vi "Alladio Tool.vi"() -> ()   [LabVIEW 2021]
doc: "Aplicación para evaluación de aparatos que usen el protocolo GEA2."
uses:
  Common/LabVIEW GEA2 Toolkit/GEA3/type defs/Data In.ctl
  Common/LabVIEW GEA2 Toolkit/GEA3/type defs/Source_Destination.ctl
  Common/LabVIEW GEA2 Toolkit/GEA3/type defs/ERD Write Data In.ctl
  Common/LabVIEW GEA2 Toolkit/GEA3/type defs/Data Type.ctl
  Common/LabVIEW GEA2 Toolkit/GEA3/type defs/ERD Read Data Out.ctl
  Common/LabVIEW GEA2 Toolkit/GEA3/type defs/ERD Read Data In.ctl
  Common/type defs/Programming.ctl
  Common/type defs/Flash_Results.ctl
  Common/type defs/ERDList.ctl
  Common/type defs/ERD_Loop_States.ctl
  Common/type defs/Version.ctl
  Common/type defs/BootloaderVersion.ctl
  Common/LabVIEW GEA2 Toolkit/GEA3/type defs/Data Out.ctl
  Alladio Tool Suport/Type defs/ERD_Always_Show_ARG.ctl
  Alladio Tool Suport/Type defs/Data_In_Automation_Bootloader.ctl
  Alladio Tool Suport/Type defs/Table_Result_Automation_BootLoader.ctl
  Alladio Tool Suport/Automation Erds/AT_Erd_Sequence.ctl
  Alladio Tool Suport/Automation Erds/Table_Result_AT_Test.ctl
  Alladio Tool Suport/Automation Erds/AT_Sequennce_Select.ctl
  D:/Common/LabVIEW GEA2 Toolkit/source/GEA3 DLL Source/GeaCommunication.dll
  Common/LabVIEW GEA2 Toolkit/source/GEA3 DLL Source/GeaCommunication.dll
  Common/GExplorer Support/typedefs/GExplorer_Data_Cluster.ctl
  Common/type defs/ERD_Data_Loop_Control.ctl
  Common/type defs/Error_Command.ctl
  Common/type defs/Cont_Send_States.ctl
  Alladio Tool Suport/Type defs/All_Bundled_Data_ARG.ctl
  Common/type defs/CSV_File_String_Arrays.ctl
  Common/type defs/Fault Table Array.ctl
  Common/type defs/Fault_Table_Info.ctl
  Common/type defs/ERD_Loop_Control_Command.ctl
  Common/type defs/GEA2_Control_Command.ctl
  Common/LabVIEW GEA2 Toolkit/GEA3/advanced/GEA2 Message Received Event Handler.vi
  Common/LabVIEW GEA2 Toolkit/GEA3/library/GEA2_Toolkit.lvlib
panel:
  out "UI LEDS":T1
  out "ERD_Always Show":T2
  out "Message":string
  in  "EndOfCycle":bool
  in  "Board Index":u8=1 min=1 max=10 step=1
  in  "Pause(mls)":u32=100
  out "Rate":u32=100
  out "State":T3=enum."Read ERDs"
  in  "Data ON":bool=TRUE
  in  "Stop":bool
  in  "Reset":bool
  in  "Tab Control":T4(tab)=enum."Log/Programming"
  out "Personality Set":u8=1
  in  "?":u8=1
  in  "Set Personality":bool
  out "CSV File Log Path":path=path "D:/QA/Commercial 2/Dryer_Xolo/ProbandoC2_24-11-21_15-05-37.csv"
  out "Version":T5
  in  "Read ERD List":T6[](array[typedef])=[{"ERD Number"=49, "Data Type"=enum."string"}] {"ERD Number" format="%.0x"}
  in  "Read ERD":bool
  in  "Write ERD List":T7[](array[typedef])=[{"ERD Number"=49, "Data Type"=enum."string", "Data"="01"}] {"ERD Number" format="%.0x"}
  in  "Write ERD":bool
  out "Read ERD Data Out":T9[](array[typedef])=[{"ERD Number"=49, "Data"="00 00 00 16"}] {"ERD Number" format="%.0x"}
  out "Boot Loader Version":T10
  in  "GEA Inputs":T11={"Source"=229, "Destination"=192} {"Destination" format="%.0x"; "Source" format="%.0x"}
  out "ERD's de Usuario":T12
  in  "Json File Path":path
  out "ERD Out Json":cluster{"ERD Number":u16, "Data":string}[](array[cluster]) {"ERD Number" format="%.0x"}
  out "Converted Data Out":T13 {"CRC" format="%04x"; "Length" format="%02x"; "Command" format="%02x"; "Destination" format="%02x"; "Source" format="%02x"}
  in  "Send Button":bool
  in  "GEA2 Send":T14={"Source"=228, "Destination"=192, "Command"=0, "Message"=""} {"Command" format="%02x"; "Destination" format="%02x"; "Source" format="%02x"}
  in  "Exit Botloader":bool
  in  "Enum":enum16{"All", "MC", "UI"}(ring)
  in  "Entry Botloader":bool
  out "OK?":bool
  in  "Parametric":T15(ring)
  in  "Write parametric":bool
  in  "Message to send":string="04 03"
  in  "Array":T16[](array[typedef]) {"Command" format="%02x"; "Destination" format="%02x"; "Source" format="%02x"}
  in  "Start_BootLoader":bool
  out "Bootloader Results":T17
  out "GEA2 Log":string
  in  "Save Log":bool
  in  "GEA2 Log Length":i32=100000
  in  "Clear":bool
  in  "Programming":T18={"Program"=FALSE, "File Path"=path "", "Program Ind"=FALSE, "Reset Board"=FALSE, "Enter Bootloader"=FALSE, "Result"=9} {"Result" items=["ImageRejected", "BoardNotFound", "UnableToGetGeaConfiguration", "WriteToFlashNotAllowed", "ImageDownloadedSuccessfully", "ImagePresent", "WriteToFlashFailed", "EraseFailed", "CrcFailed", ""]}
  in  "ERD Default List":T20=[{"Boolean"=TRUE, "ERD Number"=1792, "ERD Nanme"="Erd_ResetCount", "Data_Type"=enum."string"}, {"Boolean"=TRUE, "ERD Number"=61467, "ERD Nanme"="Erd_MabeCommunicationRequest1Data ", "Data_Type"=enum."string"}] {"ERD Number" format="%x"}
  in  "ERD's List Ticket Testing":T20 {"ERD Number" format="%x"}
  in  "Start_Test":bool
  in  "#Executions":i32=1 min=1 step=1
  in  "Array_Test":T21 {"Time to Wait (ms)" min=100; "ERD Number" format="%.0x"}
  in  "Sequence Select":T22
  in  "Save_Auto":bool
  out "Resultados AT Test":T23
  in  "Wifi State":T24(ring)
  in  "Set Wifi State(ERD 6003)":bool
  in  "Turn on Wifi":bool
  in  "Turn off Wifi":bool
  out "Wifi Network State":string
  out "Wifi Password":string
  out "Wifi Network Name":string
  out "Mac Address":string
  in  "Get Wifi Data":bool
  out "Error Out":errorcluster
  # "Personality"
  # "Ver. 0.1"
  # "Los primeros 10 ERD's apareceran\nen los indicadores de la página \nde GEA2"
  # "Wifi State is Writing to ERD 6003 and communicating with the wifi board directly.  It will remain in the state you wrote it to until another command is recieved. \n\nOnly Write to invalid if you are testing the board in Invalid state."
  # "After turning on Wifi , wait about 30 seconds and press the Get Wifi Data button.  Network state should be 1, apmode.\n\nAll this is doing is Writing the ERD 0xF115 Service Request to request connect, or disconnect."
  # "Contact:\n\nLeonel Nieto\nleonel.nieto@mabe.com.mx"
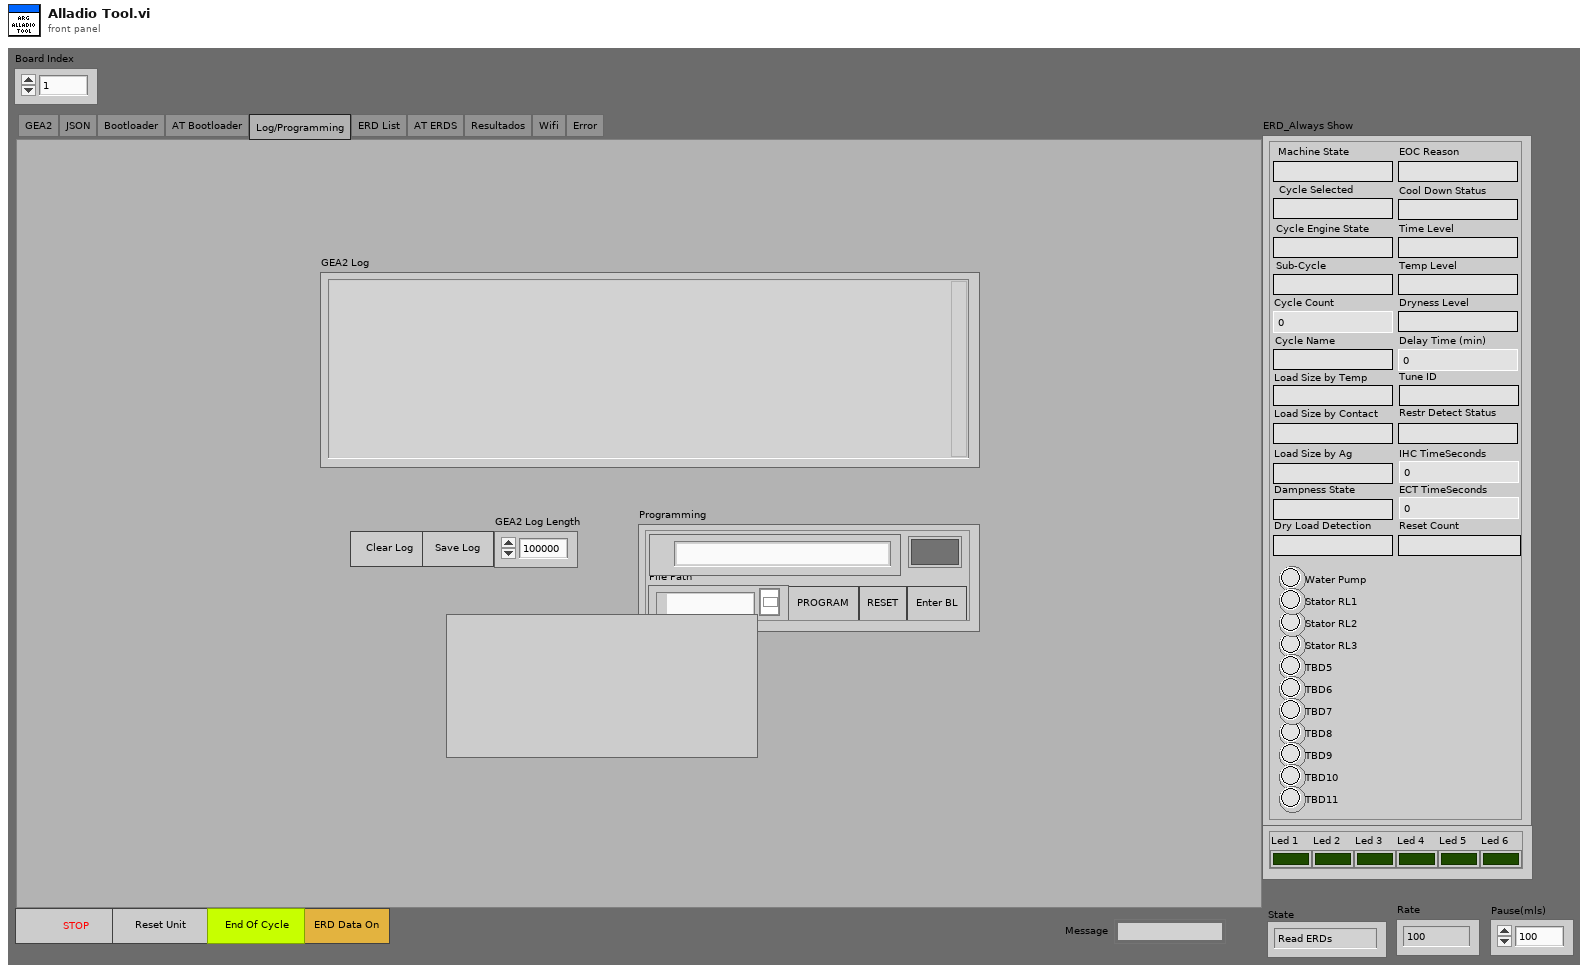
[diagram p1: front panel]
types:
  T1 = cluster{"Led 1":bool, "Led 2":bool, "Led 3":bool, "Led 4":bool, "Led 5":bool, "Led 6":bool}
  T2 = typedef "ERD_Always_Show_ARG.ctl" = cluster{"Machine State":string, "Cycle Selected":string, "Cycle Engine State":string, "Cycle Count":u32, "Temp Level":string, "Dryness Level":string, "Time Level":string, "Delay Time (min)":u16, "Sub-Cycle":string, "Cycle Name":string, "Tune ID":string, "Restr Detect Status":string, "Load Size by Contact":string, "Load Size by Temp":string, "EOC Reason":string, "Reset Count":string, "Dampness State":string, "Stator RL3":bool, "TBD5":bool, "TBD6":bool, "Water Pump":bool, "Stator RL2":bool, "Cool Down Status":string, "TBD8":bool, "TBD9":bool, "TBD10":bool, "TBD11":bool, "TBD7":bool, "Stator RL1":bool, "IHC TimeSeconds":u32, "ECT TimeSeconds ":u32, "Load Size by Ag":string, "Dry Load Detection":string}
  T3 = typedef "ERD_Loop_States.ctl" = enum16{"Init", "Build ERD Read List", "Read ERDs", "Get Version", "ERD´s User show", "Update UI", "Read Faults", "Log Data", "Pause", "Shutdown"}
  T4 = enum32{"GEA2", "JSON", "Bootloader", "AT Bootloader", "Log/Programming", "ERD List", "AT ERDS", "Resultados", "Wifi", "Error"}
  T5 = typedef "Version.ctl" = cluster{"Build Number":string, "Build Hash ":string, "Application Version":string, "Parametric Version":string, "UI App Version":string}
  T6 = typedef "ERD Read Data In.ctl" = cluster{"ERD Number":u16, "Data Type":enum16{"string", "boolean", "uint8_t", "uint16_t", "uint32_t", "uint64_t", "int8_t", "int16_t", "int32_t", "int64_t"}}
  T7 = typedef "ERD Write Data In.ctl" = cluster{"ERD Number":u16, "Data Type":T8, "Data":string}
  T8 = typedef "Data Type.ctl" = enum16{"string", "boolean", "uint8_t", "uint16_t", "uint32_t", "uint64_t", "int8_t", "int16_t", "int32_t", "int64_t"}
  T9 = typedef "ERD Read Data Out.ctl" = cluster{"ERD Number":u16, "Data":string}
  T10 = typedef "BootloaderVersion.ctl" = cluster{"UI BL Version":string, "MC BL Version":string}
  T11 = typedef "Source_Destination.ctl" = cluster{"Source":u8, "Destination":u8}
  T12 = cluster{"[0]":string, "[1]":string, "[2]":string, "[3]":string, "[4]":string, "[5]":string, "[6]":string, "[7]":string, "[8]":string, "[9]":string}
  T13 = typedef "Data Out.ctl" = cluster{"Source":u8, "Destination":u8, "Command":u8, "Length":u8, "CRC":u16, "Message":string}
  T14 = typedef "Data In.ctl" = cluster{"Source":u8, "Destination":u8, "Command":u8, "Message":string}
  T15 = enum16{"Board SKU", "Board Serial Number", "Unit SKU", "Unit Serial Number"}
  T16 = typedef "Data_In_Automation_Bootloader.ctl" = cluster{"Source":u8, "Destination":u8, "Command":u8, "Message":string, "Expected Data":string}
  T17 = typedef "Table_Result_Automation_BootLoader.ctl" = string[][]
  T18 = typedef "Programming.ctl" = cluster{"Program":bool, "File Path":path, "Program Ind":bool, "Reset Board":bool, "Enter Bootloader":bool, "Result":T19}
  T19 = typedef "Flash_Results.ctl" = i32
  T20 = typedef "ERDList.ctl" = cluster{"Boolean":bool, "ERD Number":u16, "ERD Nanme":string, "Data_Type":enum16{"string", "boolean", "uint8_t", "uint16_t", "uint32_t", "uint64_t", "int8_t", "int16_t", "int32_t", "int64_t"}}[]
  T21 = typedef "AT_Erd_Sequence.ctl" = cluster{"Accion":string, "Valor Esperado":string, "ERD Number":u16, "Data_To_Write":string, "Time to Wait (ms)":u32}[]
  T22 = typedef "AT_Sequennce_Select.ctl" = enum16{"Manual", "T361"}
  T23 = typedef "Table_Result_AT_Test.ctl" = string[][]
  T24 = enum16{"0 - OFF", "1 - App Mode", "2 - Connecting", "3 - Connected", "4 - Connected Off", "5 - Scanning", "6 - Reconnecting", "255 - Invalid"}
  T25 = typedef "All_Bundled_Data_ARG.ctl" = cluster{"Version":T5, "Personality Set":u8, "CSV File String Arrays":T26, "Fault Table Array ":T27, "ERD_Always Show":T2, "UI LEDS":cluster{"Led 1":bool, "Led 2":bool, "Led 3":bool, "Led 4":bool, "Led 5":bool, "Led 6":bool}, "Boot Loader Version":T10}
  T26 = typedef "CSV_File_String_Arrays.ctl" = cluster{"ERD Number Array":string[], "ERD Name Array":string[], "ERD Converted String Data":string[]}
  T27 = typedef "Fault Table Array.ctl" = T28[]
  T28 = typedef "Fault_Table_Info.ctl" = cluster{"Cycle Count":u32, " Runtime (min) ":u32, "Fault Status":string, "Fault ID":string, "Fault Count":u16}
  T29 = typedef "Cont_Send_States.ctl" = enum16{"Run", "Shutdown"}
  T30 = typedef "ERD_Data_Loop_Control.ctl" = cluster{"Data":variant, "State":T3}
  T31 = typedef "Error_Command.ctl" = enum16{"Initialize", "Handle Errors", "Report Errors"}
  T32 = typedef "GExplorer_Data_Cluster.ctl" = cluster{"Data":variant, "State":enum16{"Add to Log", "Clear", "Shutdown"}}
  T33 = enum8{"Enabled", "Disabled", "Disabled and Grayed Out"}
  T34 = typedef "GEA2_Control_Command.ctl" = enum16{"Initialize", "Shutdown"}
  T35 = typedef "ERD_Loop_Control_Command.ctl" = enum16{"Initialize", "Shutdown"}
  T36 = typedef "ERD_Loop_States_JL.ctl" = enum16{"Init", "Build ERD Read List", "Read ERDs", "Get Version", "ERD´s User show", "Update UI", "Read Faults", "Log Data", "Pause", "Shutdown"}
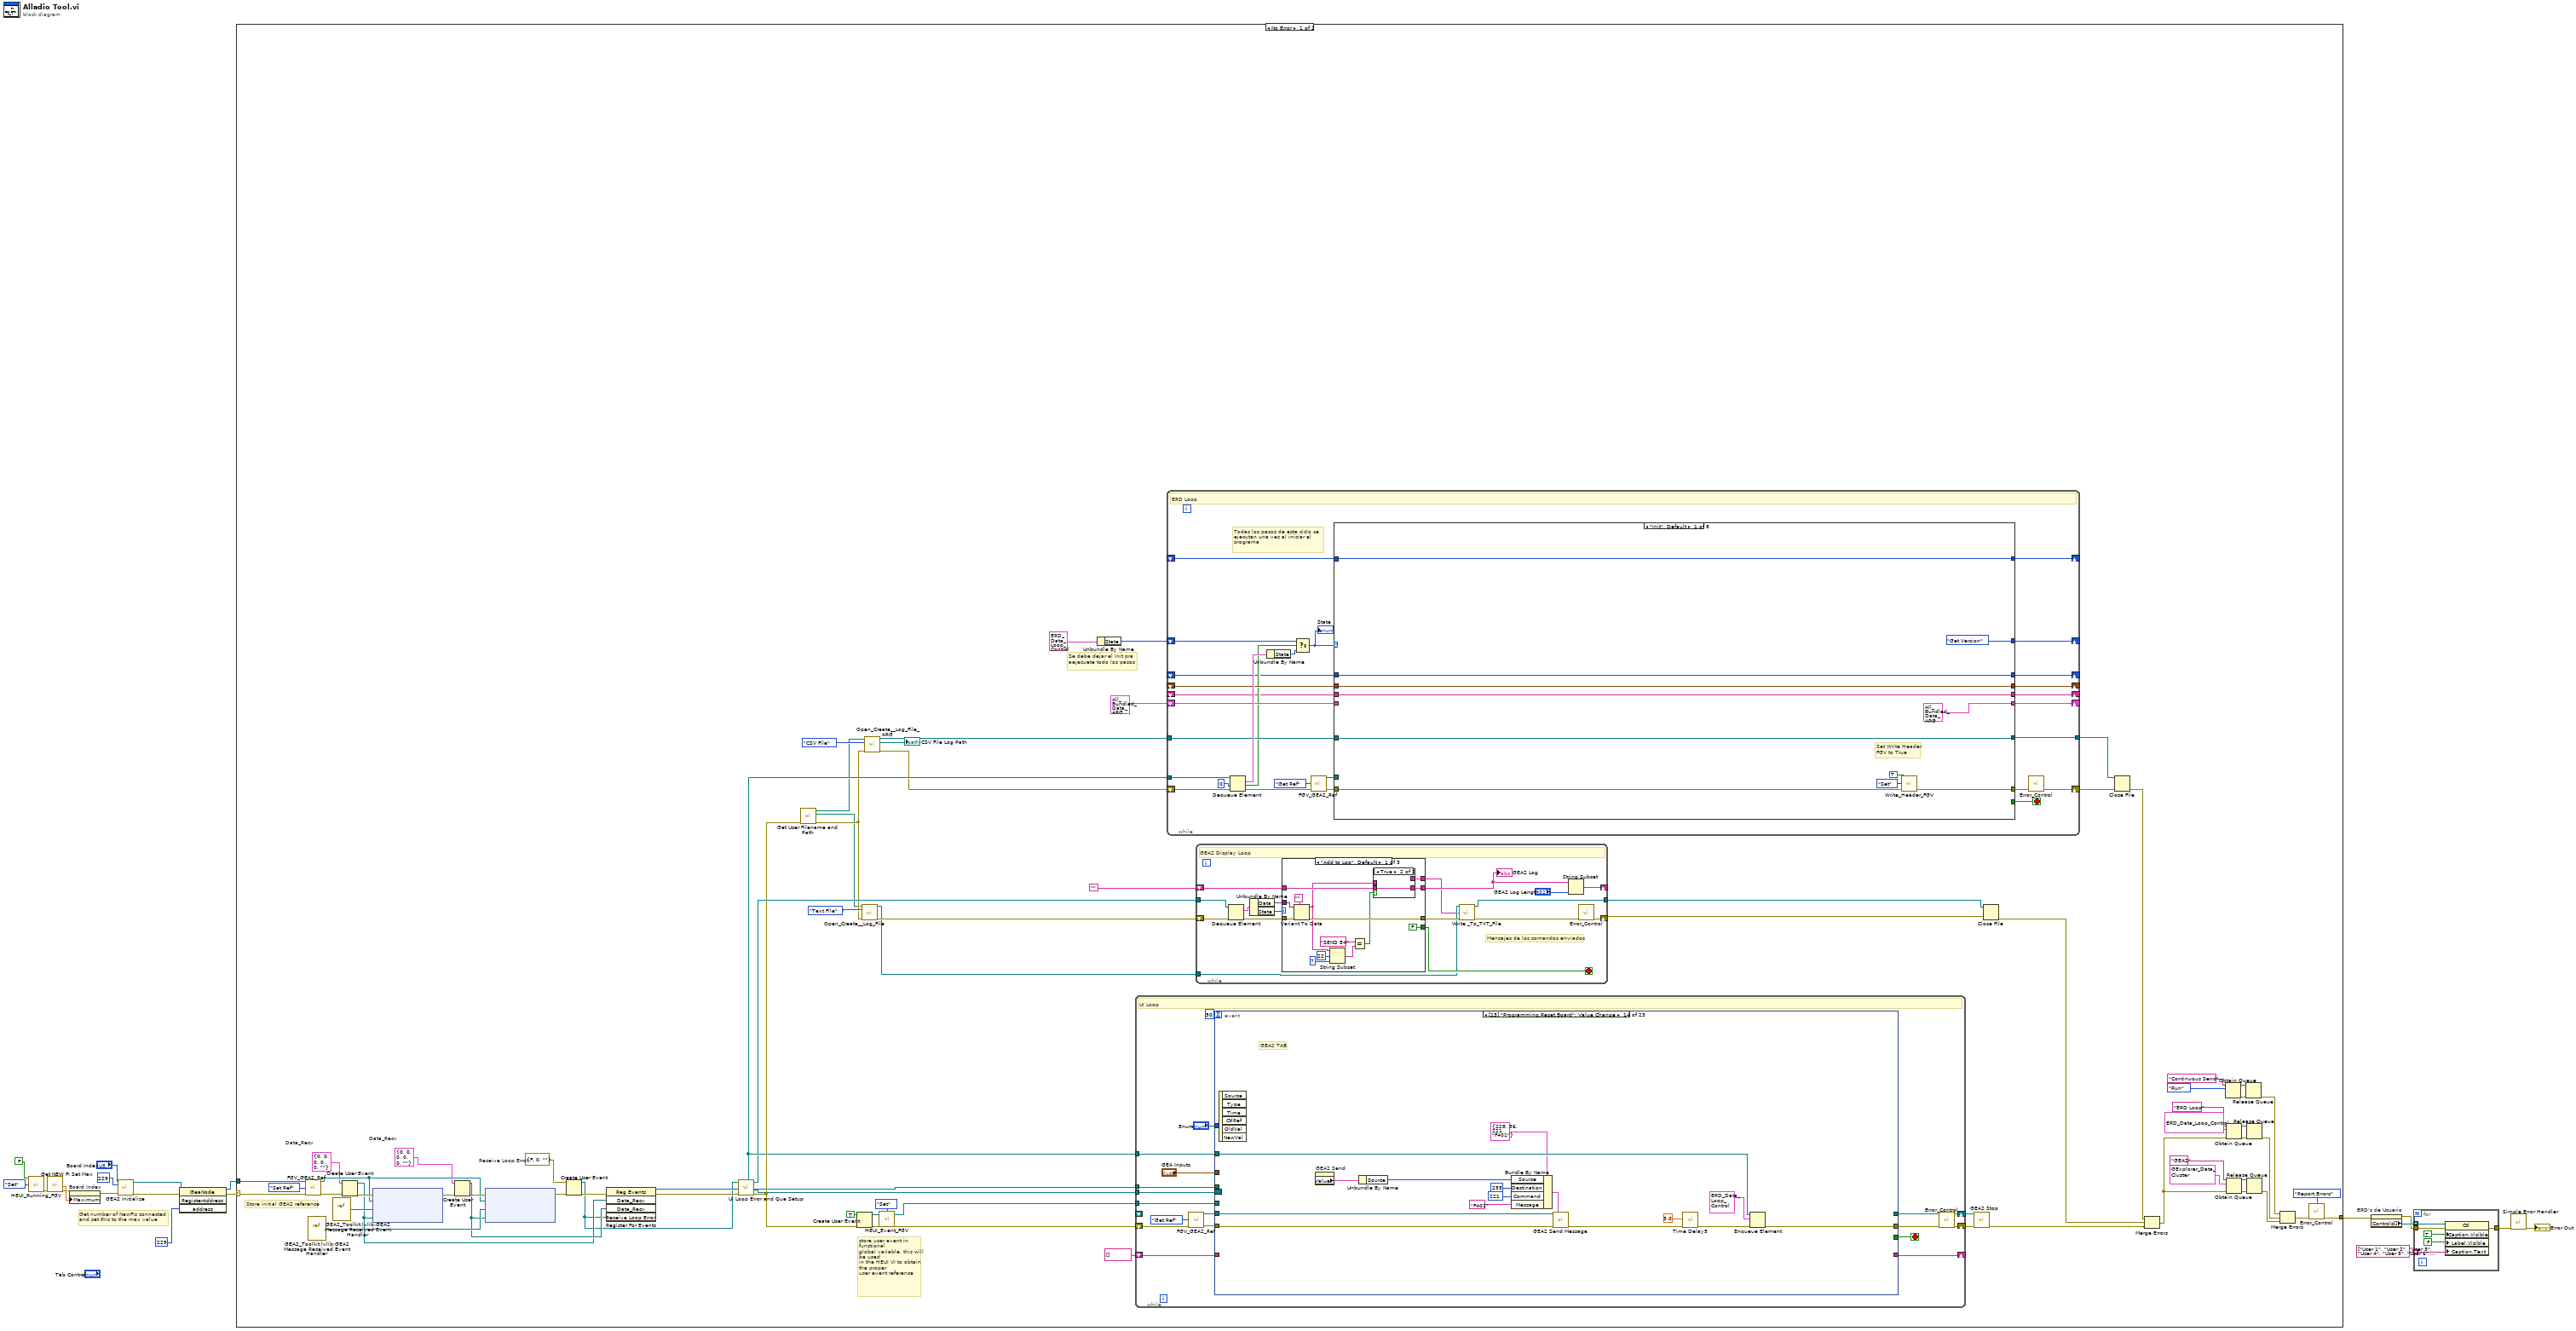
[diagram p0: block diagram]
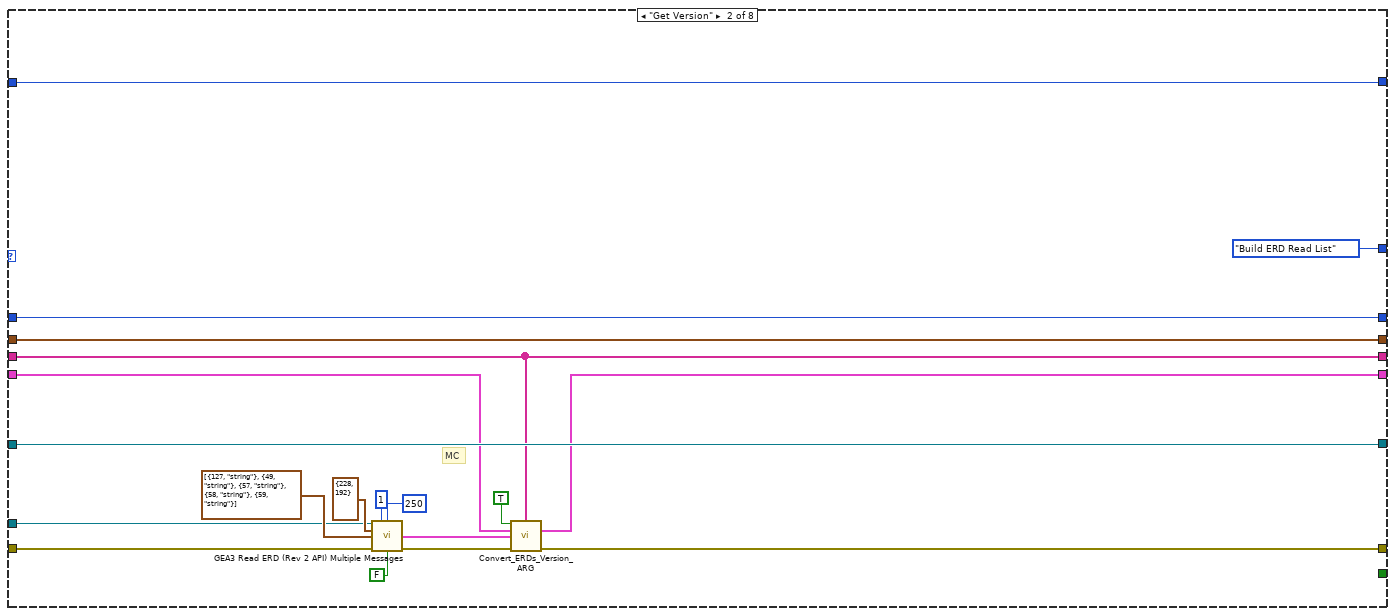
[diagram p2: hidden frame]
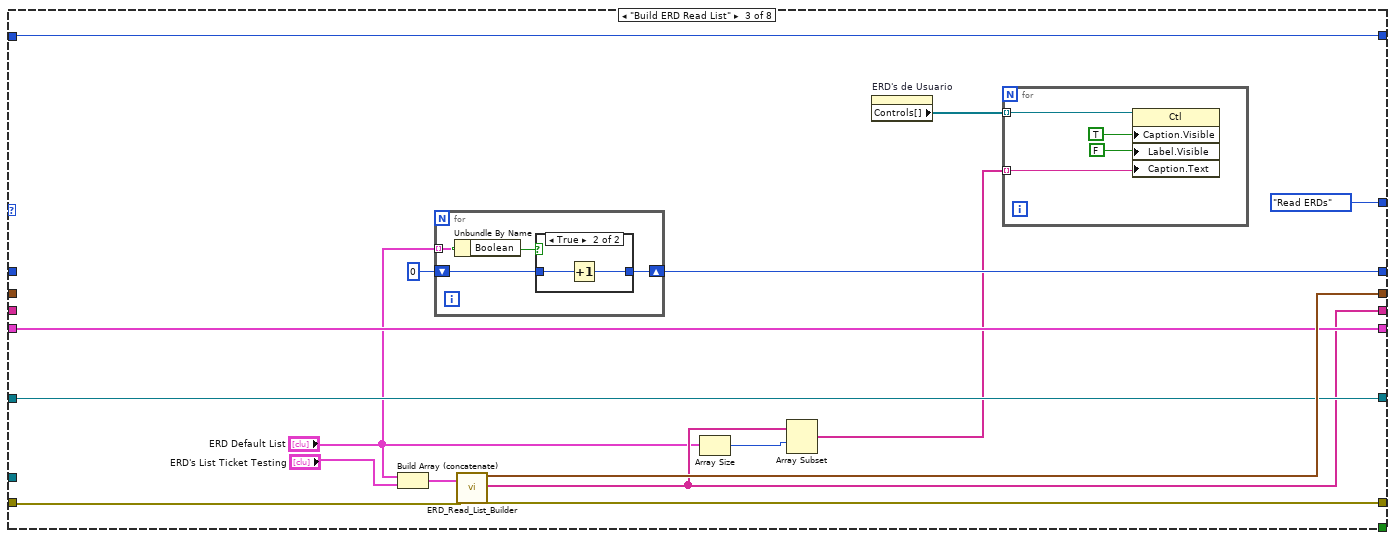
[diagram p3: hidden frame]
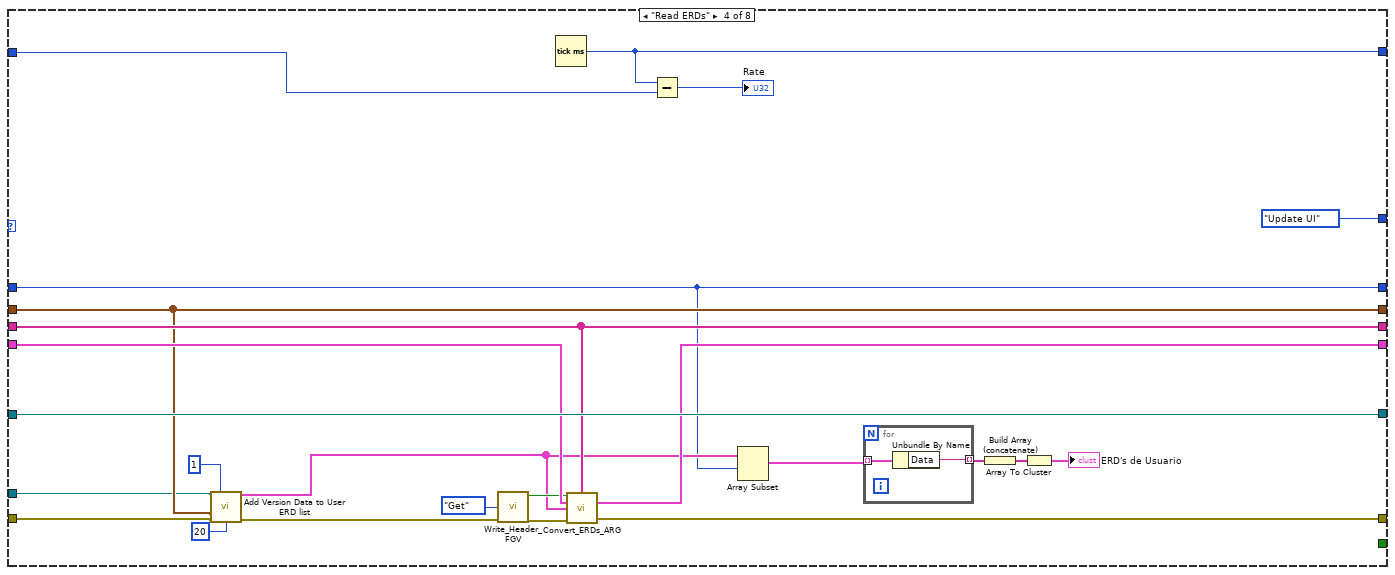
[diagram p5: hidden frame]
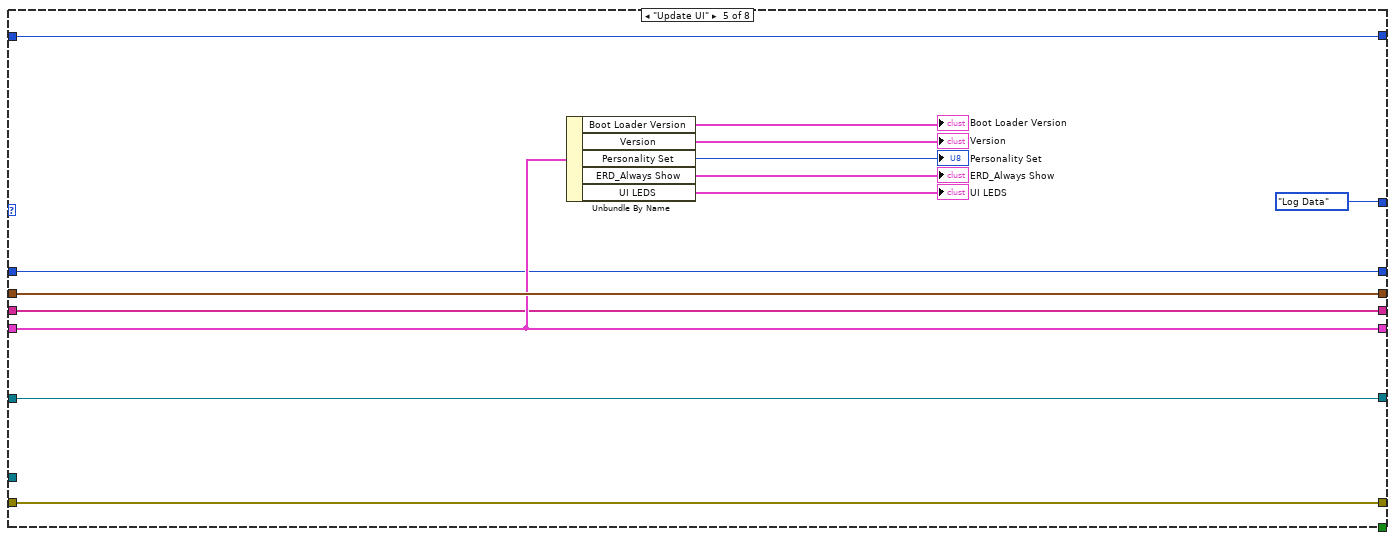
[diagram p6: hidden frame]
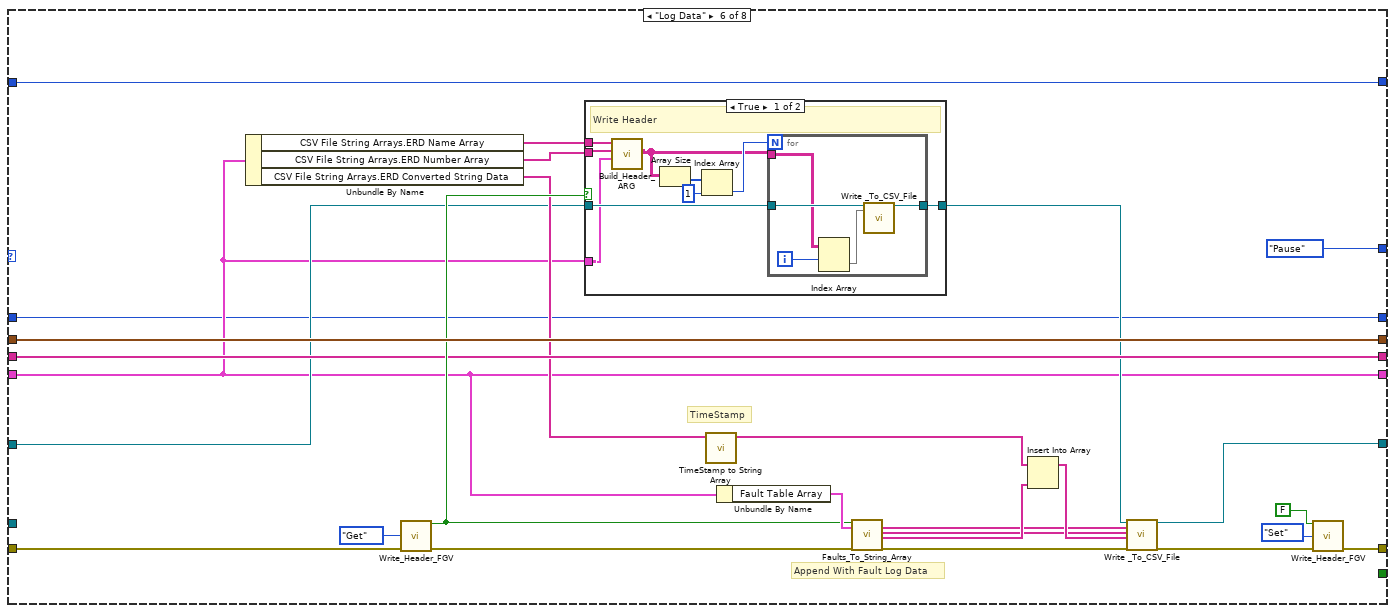
[diagram p7: hidden frame]
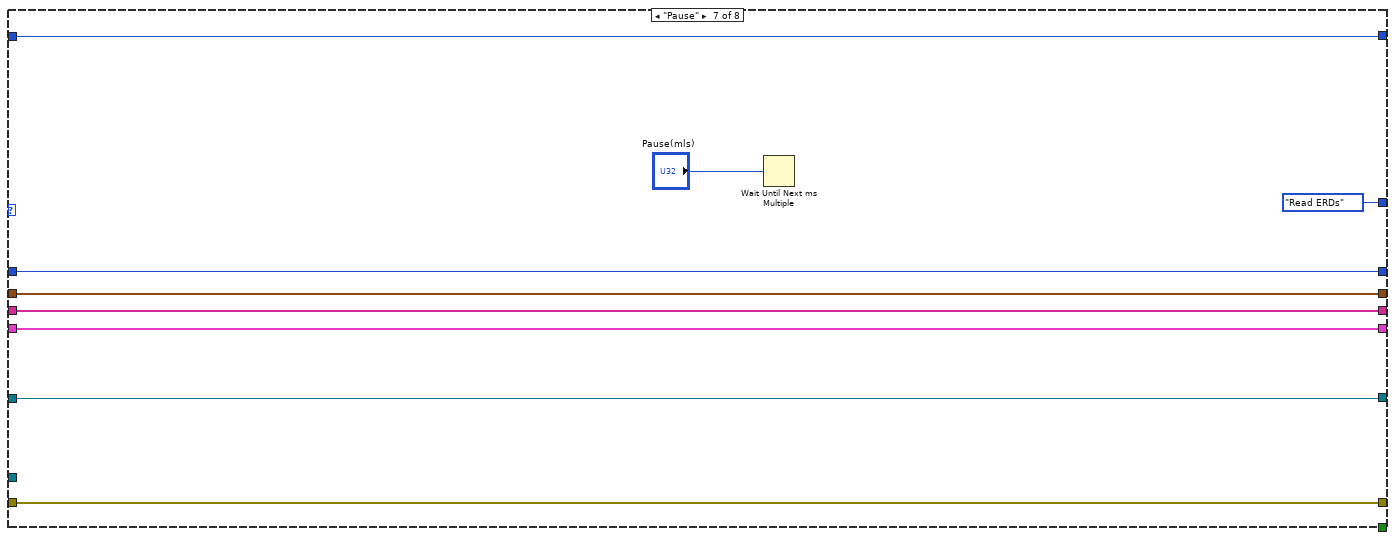
[diagram p9: hidden frame]
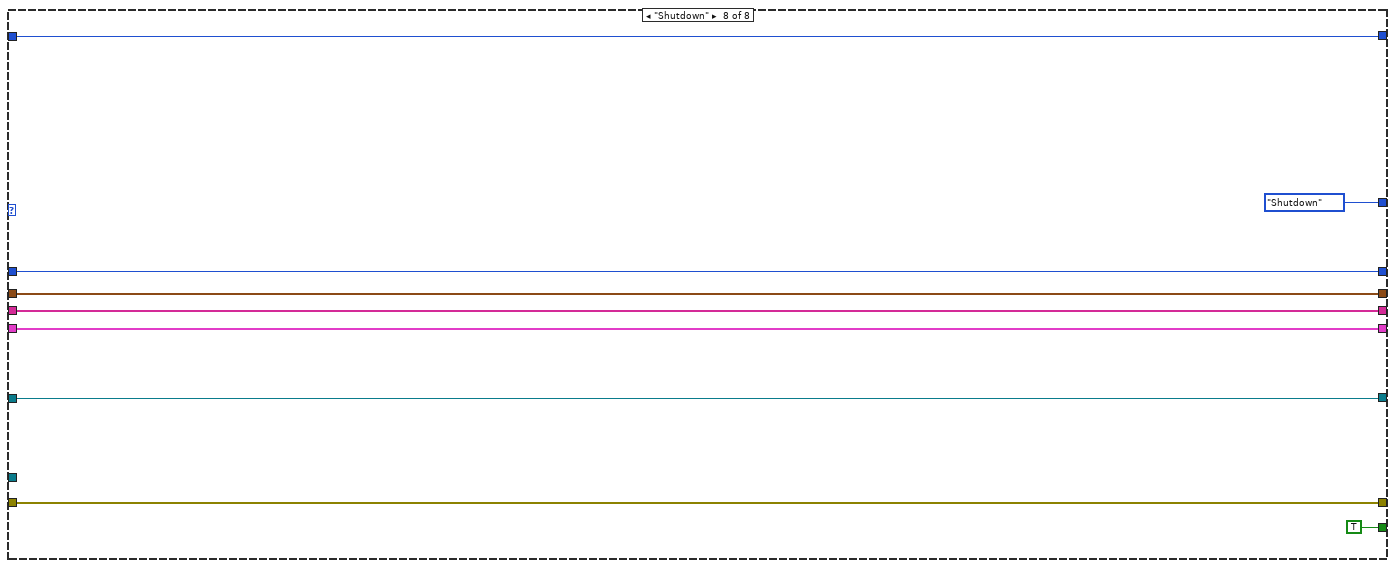
[diagram p10: hidden frame]
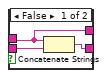
[diagram p11: hidden frame]
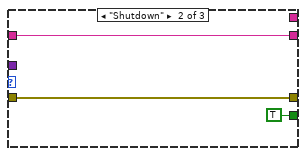
[diagram p12: hidden frame]
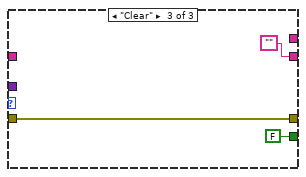
[diagram p13: hidden frame]
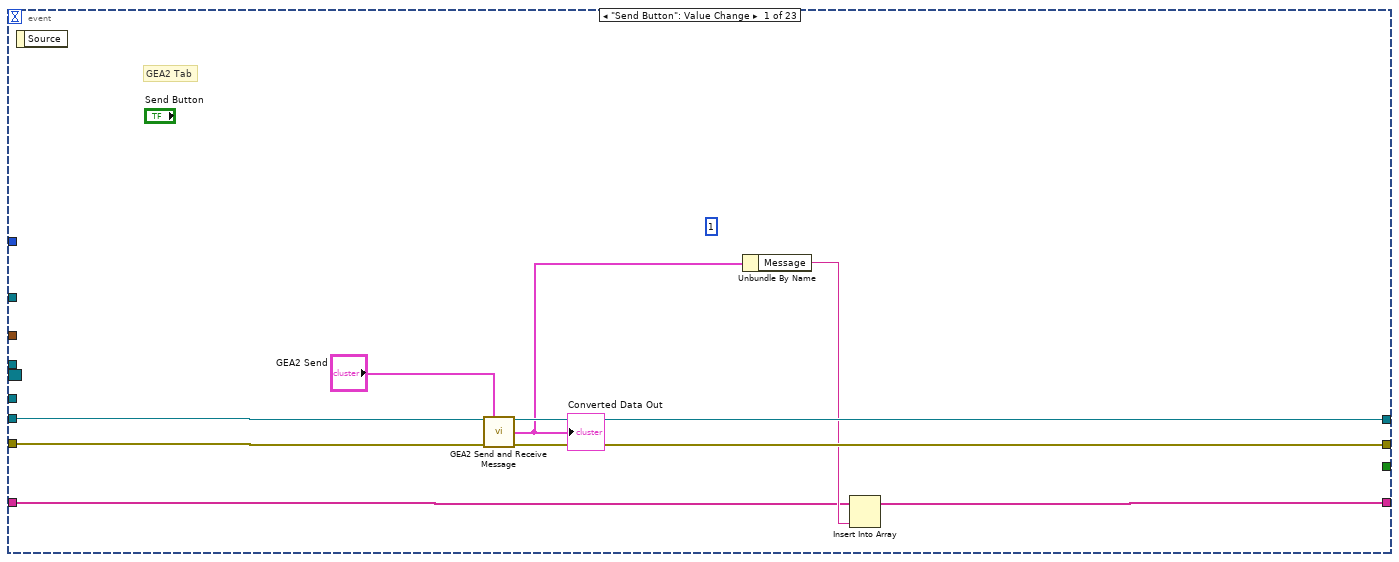
[diagram p14: hidden frame]
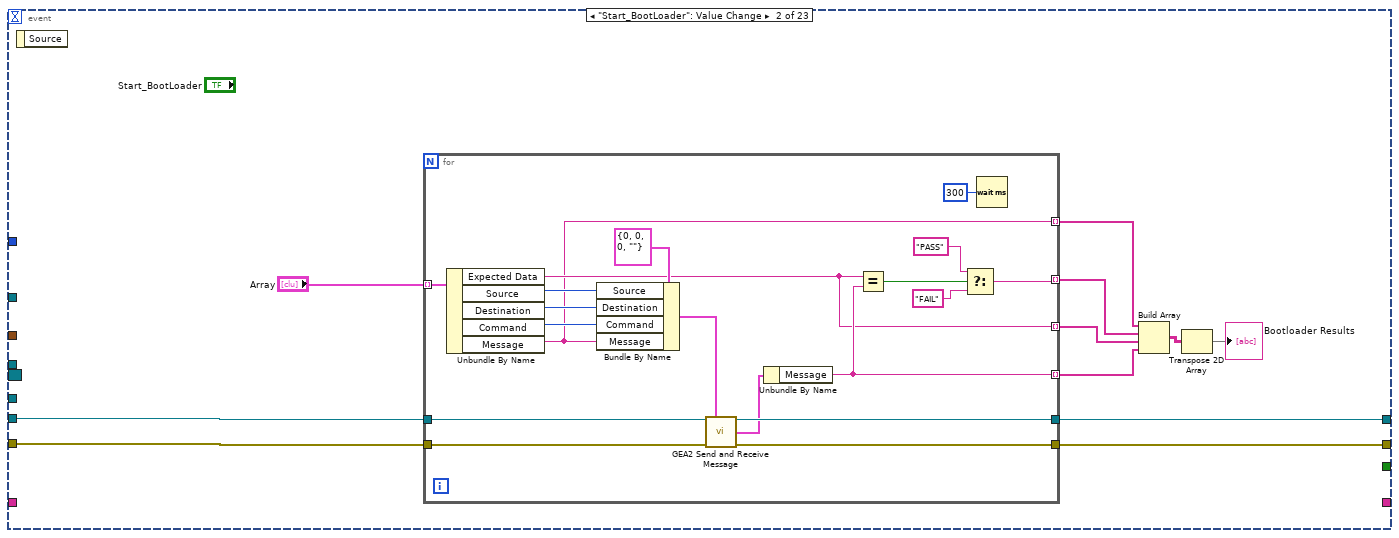
[diagram p15: hidden frame]
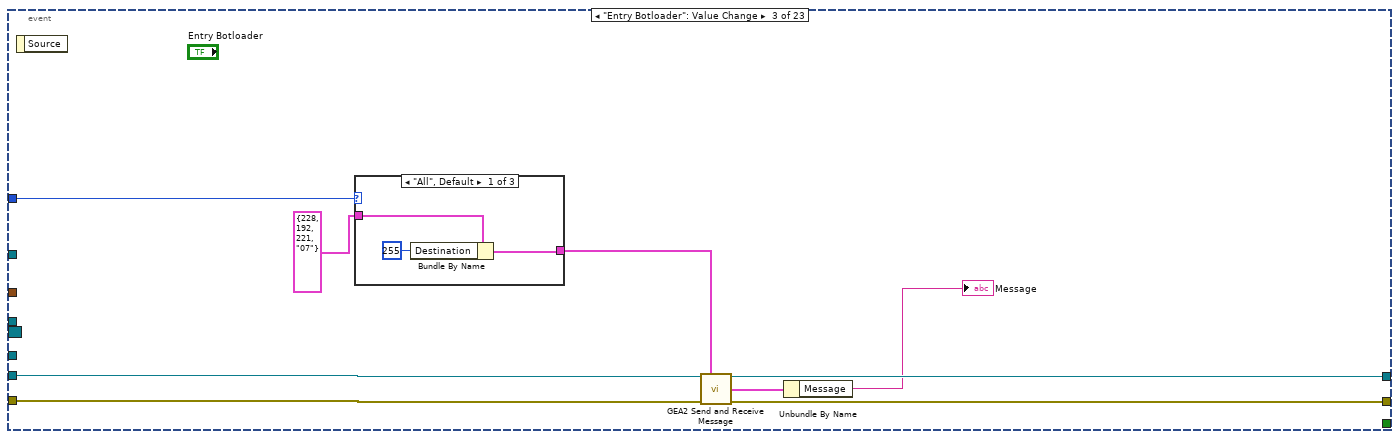
[diagram p16: hidden frame]
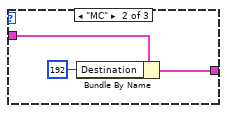
[diagram p17: hidden frame]
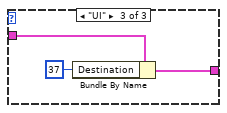
[diagram p18: hidden frame]
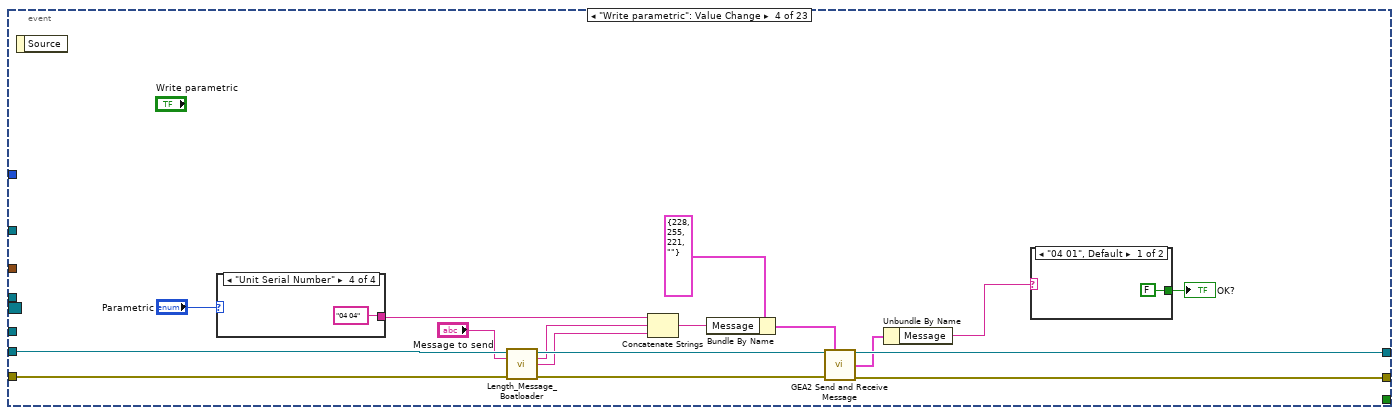
[diagram p19: hidden frame]
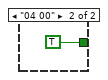
[diagram p20: hidden frame]
diagram:
  # "Get number of NewFIs connected\nand set this to the max value"
  n1 = call "HEUI_Running_FGV.vi"("Running?"=FALSE, "Action"=enum16{"Get", "Set"}."Set") -> ("Error Out"=w19:errorcluster)  [unwired: 12 in, 1 out]
  n2 = call "Get NEW FI Set Max.vi"("error in (no error)"=w19) -> ("Error Out"=w14:errorcluster, "Get Max_Out"=w15:dbl)  [unwired: 9 in]
  n3 = property on="Board Index" class="DigNum (strict)"(error in=w14, "Maximum"=w15) -> (error out=w13:errorcluster)  [unwired: 1 in, 1 out]
  n4 = call "GEA2 Initialize.vi"("Board Index"="Board Index", "Source Address"=u8 229, "error in"=w13) -> ("GEA2 Reference Out"=w11:refnum<k24>, "error out"=w8:errorcluster)  [unwired: 10 in, 1 out]
  n5 = invoke class="GeaNode" method="RegisterAddress"(reference=w11, error in=w8, "address"=u8 229 ("Source Address")) -> (reference out=w9:refnum<k24>, error out=w10:errorcluster)  [unwired: 1 in, 2 out]
  n6 = case shown="No Error" w10 {
    selector: w10 -> [w75 w719]
    tunnel: [w76 w719] -> w2
    tunnel: w9 -> [w50 _]
    frame No Error {
      w31 = T13 {"Source"=0, "Destination"=0, "Command"=0, "Length"=0, "CRC"=0, "Message"=""}  # Data_Recv
      w33 = T13 {"Source"=0, "Destination"=0, "Command"=0, "Length"=0, "CRC"=0, "Message"=""}  # Data_Recv
      w41 = errorcluster {"status"=FALSE, "code"=0, "source"=""}  # Receive Loop Error
      # "Se debe dejar el Init pra aejecuete todo los pasos"
      # "store user event in functional\nglobal variable, this will be used\nin the HEUI VI to obtain the proper\nuser event reference"
      # "Store initial GEA2 reference"
      n7 = call "FGV_GEA2_Ref.vi"("GEA2 Reference In"=w50, "Action"=enum16{"Set Ref", "Get Ref"}."Set Ref", "Error In"=w75) -> ("GEA2 Reference Out"=w44:refnum<k24>, "Error Out"=w32:errorcluster)  [unwired: 11 in]
      n8 = vi-ref "GEA2_Toolkit.lvlib:GEA2 Message Received Event Handler.vi"() -> (w42:refnum<vi>)
      n9 = vi-ref "GEA2_Toolkit.lvlib:GEA2 Message Received Event Handler.vi"() -> (w43:refnum<vi>)
      n10 = Create User Event(user event datatype=w33, error in=w32) -> (user event=w37:refnum<user-event>, error out=w46:errorcluster)
      n11 = node(w46, w44, w43, w37) -> (w47:errorcluster)  [unwired: 1 in, 1 out]
      n12 = Create User Event(user event datatype=w31, error in=w47) -> (user event=w38:refnum<user-event>, error out=w45:errorcluster)
      n13 = node(w45, w44, w42, w38) -> (w40:errorcluster)  [unwired: 1 in, 1 out]
      n14 = Create User Event(user event datatype=w41, error in=w40) -> (user event=w34:refnum<user-event>, error out=w39:errorcluster)
      n15 = register-events(error in=w39, w37, w38, w34) -> (reference out=w36:refnum<event-registration>, error out=w35:errorcluster)  [unwired: 1 in]
      n16 = call "UI Loop Error and Que Setup.vi"("error in (no error)"=w35, "Receive Loop"=w34) -> ("error out"=w23:errorcluster, "UI Loop Event Registration"=w49:refnum<event-registration>, "GEA Display Queue"=w51:refnum<queue>, "ERD Queue Loop"=w52:refnum<queue>)  [unwired: 6 in]
      n17 = call "Get User Filename and Path.vi"("error in (no error)"=w23) -> ("error out"=w22:errorcluster, "TXT File Path"=w21:path, "CSV File Path"=w20:path)  [unwired: 8 in]
      n18 = Create User Event(user event datatype=TRUE ("Bool"), error in=w23) -> (user event=w71:refnum<user-event>, error out=w72:errorcluster)
      n19 = call "Open_Create__Log_File.vi"("File Path Control"=w21, "Enum"=enum16{"CSV File", "Text File"}."Text File", "Error In"=w22) -> ("refnum out"=w56:refnum<file>, "Error Out"=w57:errorcluster)  [unwired: 10 in, 1 out]
      n20 = call "Open_Create__Log_File_ARG.vi"("File Path Control"=w20, "Enum"=enum16{"CSV File", "Text File"}."CSV File", "Error In"=w22) -> ("refnum out"=w27:refnum<file>, "File Path"=→"CSV File Log Path":path, "Error Out"=w29:errorcluster)  [unwired: 10 in]
      n21 = call "HEUI_Event_FGV.vi"("Event In"=w71, "Action"=enum16{"Get", "Set"}."Set", "Error In"=w72) -> ("Event Out"=w68:refnum<user-event>, "Error Out"=w69:errorcluster)  [unwired: 11 in]
      n22 = Unbundle By Name(T30 {"Data"=variant, "State"=enum."Init"} ("Data")) -> ("State"=w66:T3)
      n23 = while "UI Loop" {
        shift-right: [w332] -> w92
        shift-left: w69 -> [w326]
        shift-right: [w334] -> w91
        shift-left: _ -> [_]
        tunnel: w49 -> [w333]
        tunnel: w68 -> [w323]
        tunnel: w52 -> [w322]
        tunnel: w36 -> [w321]
        shift-right: [w319] -> _
        shift-left: string[] [] -> [w318]
        stop <- w331 stop-if-true
        # "UI Loop"
        n24 = call "FGV_GEA2_Ref.vi"("Action"=enum16{"Set Ref", "Get Ref"}."Get Ref", "Error In"=w326) -> ("GEA2 Reference Out"=w325:refnum<k24>, "Error Out"=w327:errorcluster)  [unwired: 12 in]
        n25 = event shown="[13] \"Programming.Reset Board\": Value Change" {
          selector: w333 -> [_ _ _ _ _ _ _ _ _ _ _ _ _ _ _ _ _ _ _ _ _ _ _]
          dyn-events: _ -> [_ _ _ _ _ _ _ _ _ _ _ _ _ _ _ _ _ _ _ _ _ _ _]
          timeout: 50 -> [_ _ _ _ _ _ _ _ _ _ _ _ _ _ _ _ _ _ _ _ _ _ _]
          tunnel: [w340 w350 w379 w406 w415 w436 w442 w459 w472 w476 w478 w487 w522 w564 w570 w588 w591 w601 w613 w626 w629 w679 w686] -> w330
          tunnel: w327 -> [w341 w353 w381 w399 w418 w433 w440 w463 w473 w476 w482 w494 w530 w569 w580 w586 w595 w602 w618 w627 w636 w683 w688]
          tunnel: [_ _ _ _ _ _ _ _ _ _ _ _ _ _ _ _ _ _ TRUE _ _ _ _] -> w331
          tunnel: w325 -> [w342 w352 w382 w405 w417 w435 w446 w462 w474 w477 w485 w496 w531 w568 w579 w584 _ _ w620 w628 w637 w684 w687]
          tunnel: [w343 w351 w380 w407 w416 w435 _ w460 w474 w477 w479 w497 _ _ w578 w582 _ _ w620 w623 w630 w680 w685] -> w334
          tunnel: "GEA Inputs" -> [_ _ _ _ _ _ w445 w461 _ _ w484 w495 _ _ _ w583 _ _ _ _ w638 w681 _]
          tunnel: w323 -> [_ _ _ _ _ _ _ _ _ _ _ _ w527 _ _ _ _ _ _ _ _ _ _]
          tunnel: w322 -> [_ _ _ _ _ _ w441 _ _ _ _ _ w521 w563 _ w587 _ w599 w612 _ _ _ _]
          tunnel: w321 -> [_ _ _ _ _ _ _ _ _ _ _ _ _ _ _ _ _ _ _ _ _ _ _]
          tunnel: "Enum" -> [_ _ w374 _ w414 _ _ _ _ _ _ _ _ _ _ _ _ _ _ _ _ _ _]
          tunnel: [w337 _ _ _ _ _ _ _ _ w475 _ _ _ _ _ _ _ _ _ _ _ _ _] -> w319
          tunnel: w318 -> [w336 _ _ _ _ _ _ _ _ w475 _ _ _ _ _ _ _ _ _ _ _ _ _]
          event "Send Button": Value Change {
            (unwired) 1
            # "GEA2 Tab"
            n26 = event-data() -> ()  [unwired: 1 in, 1 out]
            n27 = call "GEA2 Send and Receive Message.vi"("GEA2 Reference In"=w342, "Input Data"="GEA2 Send", "Error In"=w341) -> ("GEA2 Reference Out"=w343:refnum<k24>, "Converted Data Out"=w339:T13, "Error Out"=w340:errorcluster)  [unwired: 9 in, 1 out]
            "Converted Data Out" <- w339
            n28 = Unbundle By Name(w339) -> ("Message"=w338:string)
            n29 = Insert Into Array(array=w336, new element=w338) -> (w337:string[])  [unwired: 1 in]
          }
          event "Start_BootLoader": Value Change {
            n30 = event-data() -> ()  [unwired: 1 in, 1 out]
            n31 = for {
              tunnel: "Array" -> [w372] mode=indexing
              tunnel: w353 -> [w367]
              tunnel: w352 -> [w366]
              tunnel: [w365] -> w351
              tunnel: [w364] -> w350
              tunnel: [w362] -> w346 mode=indexing
              tunnel: [w361] -> w347 mode=indexing
              tunnel: [w357] -> w348 mode=indexing
              tunnel: [w355] -> w345 mode=indexing
              n32 = Unbundle By Name(w372) -> ("Expected Data"=w361:string, "Source"=w371:u8, "Destination"=w370:u8, "Command"=w369:u8, "Message"=w355:string)
              n33 = Bundle By Name(cluster=T14 {"Source"=0, "Destination"=0, "Command"=0, "Message"=""} ("Input Data"), "Source"=w371, "Destination"=w370, "Command"=w369, "Message"=w355) -> (w368:T14)
              n34 = call "GEA2 Send and Receive Message.vi"("GEA2 Reference In"=w366, "Input Data"=w368, "Error In"=w367) -> ("GEA2 Reference Out"=w365:refnum<k24>, "Converted Data Out"=w363:T13, "Error Out"=w364:errorcluster)  [unwired: 9 in, 1 out]
              n35 = Unbundle By Name(w363) -> ("Message"=w362:string)
              n36 = Equal?(x=w361, y=w362) -> (x = y?=w360:bool)
              n37 = Select(t="PASS" ("Expected Data"), s=w360, f="FAIL") -> (s? t:f=w357:string)
              n38 = Wait (ms)(milliseconds to wait=u32 300) -> ()  [unwired: 1 out]
            }
            n39 = Build Array(w345, w348, w347, w346) -> (w349:string[][])
            n40 = Transpose 2D Array(2D array=w349) -> (transposed array=→"Bootloader Results":string[][])
          }
          event "Entry Botloader": Value Change {
            n41 = event-data() -> ()  [unwired: 1 in, 1 out]
            n42 = case shown="\"All\", Default" w374 {
              tunnel: T14 {"Source"=228, "Destination"=192, "Command"=221, "Message"="07"} ("GEA2 Send") -> [w384 w388 w389]
              tunnel: [w383 w386 w390] -> w375
              frame "All", Default {
                n43 = Bundle By Name(cluster=w384, "Destination"=u8 255) -> (w383:T14)
              }
              frame "MC" {
                n44 = Bundle By Name(cluster=w388, "Destination"=u8 192) -> (w386:T14)
              }
              frame "UI" {
                n45 = Bundle By Name(cluster=w389, "Destination"=u8 37) -> (w390:T14)
              }
            }
            n46 = call "GEA2 Send and Receive Message.vi"("GEA2 Reference In"=w382, "Input Data"=w375, "Error In"=w381) -> ("GEA2 Reference Out"=w380:refnum<k24>, "Converted Data Out"=w378:T13, "Error Out"=w379:errorcluster)  [unwired: 9 in, 1 out]
            n47 = Unbundle By Name(w378) -> ("Message"=→"Message":string)
          }
          event "Write parametric": Value Change {
            n48 = event-data() -> ()  [unwired: 1 in, 1 out]
            n49 = case shown="\"Unit Serial Number\"" "Parametric" {
              tunnel: ["04 01" ("string") "04 02" ("string") "04 03" ("string") "04 04" ("string")] -> w403
              frame "Board SKU", Default {
              }
              frame "Board Serial Number" {
              }
              frame "Unit SKU" {
              }
              frame "Unit Serial Number" {
              }
            }
            n50 = call "Length_Message_Boatloader.vi"("string"="Message to send", "error in"=w399) -> ("hex integer string"=w401:string, "Message"=w400:string, "error out"=w398:errorcluster)  [unwired: 11 in]
            n51 = Concatenate Strings(w403, w401, w400) -> (w396:string)
            n52 = Bundle By Name(cluster=T14 {"Source"=228, "Destination"=255, "Command"=221, "Message"=""} ("GEA2 Send"), "Message"=w396) -> (w395:T14)
            n53 = call "GEA2 Send and Receive Message.vi"("GEA2 Reference In"=w405, "Input Data"=w395, "Error In"=w398) -> ("GEA2 Reference Out"=w407:refnum<k24>, "Converted Data Out"=w394:T13, "Error Out"=w406:errorcluster)  [unwired: 9 in, 1 out]
            n54 = Unbundle By Name(w394) -> ("Message"=w393:string)
            n55 = case shown="\"04 01\", Default" w393 {
              tunnel: [FALSE TRUE] -> w392
              frame "04 01", Default {
              }
              frame "04 00" {
              }
            }
            "OK?" <- w392
          }
          event "Exit Botloader": Value Change {
            n56 = event-data() -> ()  [unwired: 1 in, 1 out]
            n57 = case shown="\"All\", Default" w414 {
              tunnel: T14 {"Source"=228, "Destination"=0, "Command"=221, "Message"="F4 01"} ("GEA2 Send") -> [w422 w426 w427]
              tunnel: [w421 w424 w428] -> w419
              frame "All", Default {
                n58 = Bundle By Name(cluster=w422, "Destination"=u8 255) -> (w421:T14)
              }
              frame "MC" {
                n59 = Bundle By Name(cluster=w426, "Destination"=u8 192) -> (w424:T14)
              }
              frame "UI" {
                n60 = Bundle By Name(cluster=w427, "Destination"=u8 37) -> (w428:T14)
              }
            }
            n61 = call "GEA2 Send and Receive Message.vi"("GEA2 Reference In"=w417, "Input Data"=w419, "Error In"=w418) -> ("GEA2 Reference Out"=w416:refnum<k24>, "Error Out"=w415:errorcluster)  [unwired: 9 in, 2 out]
          }
          event "Clear": Value Change {
            w430 = T32 {"Data"=variant, "State"=enum."Clear"} ("element")
            # "GEA2 Tab"
            n62 = event-data() -> ()  [unwired: 1 in, 6 out]
            n63 = Obtain Queue(name (unnamed)="GEA2", element data type=w430, error in (no error)=w433) -> (queue out=w431:refnum<queue>, error out=w434:errorcluster)  [unwired: 2 in, 1 out]
            n64 = Enqueue Element(queue=w431, element=w430, error in (no error)=w434) -> (error out=w436:errorcluster)  [unwired: 1 in, 2 out]
          }
          event "Set Personality": Value Change {
            # "GEA2 Tab"
            n65 = event-data() -> ()  [unwired: 1 in, 6 out]
            n66 = Index Array(array=T7[] [{"ERD Number"=65281, "Data Type"=enum."string", "Data"=""}] ("Write ERD List")) -> (element=w451:T7)  [unwired: 1 in]
            n67 = Number To Hexadecimal String(1:i16 2 ("width (-)"), 2:"?") -> (0:w450:string)
            n68 = Bundle By Name(cluster=w451, "Data"=w450) -> (w449:T7)
            n69 = Build Array(w449) -> (w448:T7[])
            n70 = call "GEA2 Write ERD.vi"("GEA2 Reference In"=w446, "GEA Inputs"=w445, "Write ERD List"=w448, "Error In"=w440, "Verify ERD Response?"=TRUE) -> ("Error Out"=w438:errorcluster)  [unwired: 8 in, 2 out]
            n71 = call "Get NEW FI Set Max.vi"("error in (no error)"=w438) -> ("Error Out"=w437:errorcluster)  [unwired: 9 in, 1 out]
            n72 = call "FGV_GEA2_Ref.vi"("Action"=enum16{"Set Ref", "Get Ref"}."Get Ref", "Error In"=w437) -> ()  [unwired: 12 in, 2 out]
            n73 = Enqueue Element(queue=w441, element=T30 {"Data"=variant, "State"=enum."Init"} ("Data")) -> (error out=w442:errorcluster)  [unwired: 2 in, 2 out]
          }
          event "Start_Test": Value Change {
            n74 = event-data() -> ()  [unwired: 1 in, 1 out]
            n75 = call "AT_Sequence_Select.vi"("Array_Test"="Array_Test", "Sequence Select"="Sequence Select") -> ("Array_Test_Out"=w456:T21)  [unwired: 9 in]
            n76 = for {
              N: "#Executions" -> [_]
              tunnel: w461 -> [w468]
              tunnel: w456 -> [w467]
              shift-right: [w465] -> w459
              shift-left: w463 -> [w466]
              shift-right: [w469] -> w460
              shift-left: w462 -> [w470]
              tunnel: [w464] -> w457
              n77 = call "AT_ERDS.vi"("GEA2 Reference In"=w470, "GEA Inputs"=w468, "Array_Test"=w467, "Error In"=w466) -> ("GEA2 Reference Out"=w469:refnum<k24>, "Resultados AT Test"=w464:T23, "Error Out"=w465:errorcluster)  [unwired: 9 in]
            }
            "Resultados AT Test" <- w457
          }
          event "Save_Auto": Value Change {
            n78 = event-data() -> ()  [unwired: 1 in, 6 out]
            n79 = property on="Resultados AT Test" class="Tbl (strict)"() -> ("Value"=w471:T23)  [unwired: 2 in, 2 out]
            n80 = call "Save_Automation_Test.vi"("Resultados"=w471, "error in (no error)"=w473) -> ("error out"=w472:errorcluster)  [unwired: 13 in]
          }
          event Timeout {
            # "Must have timeout case to give GEA2 FGV a chance to update\nthe GEA2 reference. Otherwise, when we receive an event it may\nbe using a reference that is no longer valid."
            n81 = event-data() -> ()  [unwired: 1 in, 3 out]
          }
          event "Write ERD": Value Change {
            # "Read/Write ERDs Tab"
            n82 = event-data() -> ()  [unwired: 1 in, 1 out]
            n83 = call "GEA3 Write ERD (Rev 2 API) Multiple Messages.vi"("GEA2 Reference In"=w485, "# of Tries"=2 ("Retry Count"), "GEA Inputs"=w484, "Write ERD List"="Write ERD List", "Error In"=w482, "Verify ERD Response?"=TRUE) -> ("GEA2 Reference Out"=w479:refnum<k24>, "Error Out"=w478:errorcluster)  [unwired: 7 in, 1 out]
          }
          event "Read ERD": Value Change {
            # "Read/Write ERDs tab"
            n84 = event-data() -> ()  [unwired: 1 in, 6 out]
            n85 = Path To String(path="Json File Path") -> (string=w492:string)
            n86 = Empty String/Path?(string/path="Json File Path") -> ()  [unwired: 1 out]
            n87 = Match Pattern(string=w492, regular expression=".json") -> (match substring=w490:string)  [unwired: 1 in, 3 out]
            n88 = Equal?(x=".json", y=w490) -> (x = y?=w489:bool)
            n89 = case shown="True" w489 {
              tunnel: "Read ERD List" -> [w502 w519]
              tunnel: [w507 w517] -> w497
              tunnel: w496 -> [w504 w516]
              tunnel: w495 -> [w503 w515]
              tunnel: w494 -> [w505 w513]
              tunnel: "Json File Path" -> [_ w511]
              tunnel: [w506 w510] -> w487
              tunnel: [w499 w509] -> w486
              frame False {
                n90 = call "GEA3 Read ERD (Rev 2 API) Multiple Messages.vi"("GEA2 Reference In"=w504, "Retry Count"=2, "GEA Inputs"=w503, "Read ERD List"=w502, "Error In"=w505, "Verify ERD Response?"=TRUE) -> ("GEA2 Reference Out"=w507:refnum<k24>, "ERD Data Out"=w499:cluster{"ERD Number":u16, "Data":string}[], "Error Out"=w506:errorcluster)  [unwired: 6 in, 1 out]
              }
              frame True {
                n91 = call "GEA3 Read ERD (Rev 2 API) Multiple Messages.vi"("GEA2 Reference In"=w516, "Retry Count"=2, "GEA Inputs"=w515, "Read ERD List"=w519, "Error In"=w513, "Verify ERD Response?"=TRUE) -> ("GEA2 Reference Out"=w517:refnum<k24>, "ERD Data Out"=w509:cluster{"ERD Number":u16, "Data":string}[], "Error Out"=w512:errorcluster)  [unwired: 6 in, 1 out]
                n92 = call "Json_Data_Path_Argentina.vi"("Json File Path"=w511, "ERD Data In"=w509, "error in"=w512) -> ("ERD Data Out"=→"ERD Out Json":cluster{"ERD Number":u16, "Data":string}[], "error out"=w510:errorcluster)  [unwired: 11 in]
              }
            }
            "Read ERD Data Out" <- w486
          }
          event Value Change {
            (unwired) "ERD Loop" ("name (unnamed)")
            w523 = TRUE ("Blinking")
            # "GEA2 Tab"
            n93 = event-data() -> ()  [unwired: 1 in, 6 out]
            n94 = Generate User Event(user event=w527, event data cluster=TRUE ("event data"), error in=w530) -> (error out=w528:errorcluster)  [unwired: 1 in, 1 out]
            n95 = property on="Program Ind" class="Bool (strict)"(error in=w528, "Value"=w523, "Blinking"=w523) -> (error out=w524:errorcluster)  [unwired: 1 in, 1 out]
            n96 = Enqueue Element(queue=w521, element=T30 {"Data"=variant, "State"=enum."Pause"} ("Data"), error in (no error)=w524) -> (error out=w526:errorcluster)  [unwired: 1 in, 2 out]
            n97 = Unbundle By Name("Programming") -> ("File Path"=w534:path)
            n98 = call "Time Delay3"("error in (no error)"=w526, "Delay Time (s)"=2.0) -> ("error out"=w525:errorcluster)  [unwired: 9 in]
            n99 = Not Equal?(x=w534, y=path "") -> (x != y?=w533:bool)
            n100 = case shown="True" w533 {
              tunnel: w525 -> [w537 w542]
              tunnel: [w537 w549] -> w522
              tunnel: w534 -> [_ w554]
              tunnel: w531 -> [_ w550]
              frame False {
              }
              frame True {
                w540 = T19 9 items=["ImageRejected", "BoardNotFound", "UnableToGetGeaConfiguration", "WriteToFlashNotAllowed", "ImageDownloadedSuccessfully", "ImagePresent", "WriteToFlashFailed", "EraseFailed", "CrcFailed", ""] ("Result")
                w548 = FALSE ("Blinking")
                n101 = property on="Result" class="Ring (strict)"(error in=w542, "Value"=w540) -> (error out=w541:errorcluster)  [unwired: 1 in, 1 out]
                n102 = property on="Board Index" class="DigNum (strict)"(error in=w542, "DisabledEnum"=T33."Disabled and Grayed Out" ("Disabled")) -> ()  [unwired: 1 in, 2 out]
                n103 = call "GEA2 Flash APL.vi"("GEA2 Reference In"=w550, "Force Update?"=TRUE, "Source Address"=u8 228, "Destination Address"=u8 192, "File Path"=w554, "Error In"=w541, "Broadcast"=TRUE, "Reset?"=FALSE ("Reset Board?")) -> ("Result"=w543:i32, "Error Out"=w545:errorcluster)  [unwired: 3 in, 3 out]
                n104 = property on="Result" class="Ring (strict)"(error in=w545, "Value"=w543) -> (error out=w544:errorcluster)  [unwired: 1 in, 1 out]
                n105 = property on="Board Index" class="DigNum (strict)"(error in=w545, "DisabledEnum"=T33."Enabled" ("Disabled")) -> ()  [unwired: 1 in, 2 out]
                n106 = property on="Program Ind" class="Bool (strict)"(error in=w544, "Value"=w548, "Blinking"=w548) -> (error out=w549:errorcluster)  [unwired: 1 in, 1 out]
              }
            }
          }
          event Value Change {
            # "GEA2 TAB"
            n107 = event-data() -> ()  [unwired: 1 in, 6 out]
            n108 = property on="GEA2 Send" class="Clust (strict)"() -> ("Value"=w558:T14)  [unwired: 2 in, 2 out]
            n109 = Unbundle By Name(w558) -> ("Source"=w557:u8)
            n110 = Bundle By Name(cluster=T14 {"Source"=228, "Destination"=36, "Command"=221, "Message"="F401"} ("Input Data"), "Source"=w557, "Destination"=u8 255, "Command"=u8 221, "Message"="F401") -> (w561:T14)
            n111 = call "GEA2 Send Message.vi"("GEA2 Reference In"=w568, "Input Data"=w561, "Error In"=w569) -> ("Error Out"=w555:errorcluster)  [unwired: 11 in, 1 out]
            n112 = call "Time Delay5"("error in (no error)"=w555, "Delay Time (s)"=3.0) -> ("error out"=w565:errorcluster)  [unwired: 9 in]
            n113 = Enqueue Element(queue=w563, element=T30 {"Data"=variant, "State"=enum."Init"} ("Data"), error in (no error)=w565) -> (error out=w564:errorcluster)  [unwired: 1 in, 2 out]
          }
          event Value Change {
            # "GEA2 Tab"
            n114 = event-data() -> ()  [unwired: 1 in, 6 out]
            n115 = property on="GEA2 Send" class="Clust (strict)"() -> ("Value"=w577:T14)  [unwired: 2 in, 2 out]
            n116 = Unbundle By Name(w577) -> ("Source"=w573:u8, "Destination"=w572:u8)
            n117 = Bundle By Name(cluster=T14 {"Source"=228, "Destination"=36, "Command"=221, "Message"="F401"} ("Input Data"), "Source"=w573, "Destination"=w572, "Command"=u8 221, "Message"="07") -> (w571:T14)
            n118 = call "GEA2 Send Message.vi"("GEA2 Reference In"=w579, "Input Data"=w571, "Error In"=w580) -> ("GEA2 Reference Out"=w578:refnum<k24>, "Error Out"=w570:errorcluster)  [unwired: 11 in]
          }
          event "Reset": Value Change {
            # "Main"
            n119 = event-data() -> ()  [unwired: 1 in, 6 out]
            n120 = call "GEA2 Write ERD.vi"("GEA2 Reference In"=w584, "GEA Inputs"=w583, "Write ERD List"=T7[] [{"ERD Number"=50, "Data Type"=enum."string", "Data"="01"}], "Error In"=w586) -> ("GEA2 Reference Out"=w582:refnum<k24>, "Error Out"=w581:errorcluster)  [unwired: 9 in, 1 out]
            n121 = Enqueue Element(queue=w587, element=T30 {"Data"=variant, "State"=enum."Init"} ("Data"), error in (no error)=w581) -> (error out=w588:errorcluster)  [unwired: 1 in, 2 out]
          }
          event "Save Log": Value Change {
            # "GEA2 Tab"
            n122 = event-data() -> ()  [unwired: 1 in, 6 out]
            n123 = property on="GEA2 Log" class="Str"(error in=w595) -> (error out=w597:errorcluster, "Value"=w596:string)  [unwired: 1 in, 1 out]
            n124 = Write to Text File(prompt (Choose or enter file path)="Choose filename and path to save txt file to ", text=w596, error in=w597) -> (refnum out=w594:refnum<file>, error out=w593:errorcluster)  [unwired: 1 in, 1 out]
            n125 = Close File(refnum=w594, error in=w593) -> (error out=w592:errorcluster)  [unwired: 1 out]
            n126 = call <vilib>:"Clear Errors.vi"("error in (no error)"=w592, "specific error code to clear (0: all)"=43) -> ("error out"=w591:errorcluster)  [unwired: 4 in, 1 out]
          }
          event "Data ON": Value Change {
            # "Main"
            n127 = event-data() -> ()  [unwired: 1 in, 6 out]
            n128 = case shown="True" "Data ON" {
              tunnel: w602 -> [w605 w609]
              tunnel: [w604 w608] -> w601
              tunnel: w599 -> [w603 w607]
              frame True {
                n129 = Enqueue Element(queue=w603, element=T30 {"Data"=variant, "State"=enum."Init"} ("Data"), error in (no error)=w605) -> (error out=w604:errorcluster)  [unwired: 1 in, 2 out]
              }
              frame False {
                n130 = Enqueue Element(queue=w607, element=T30 {"Data"=variant, "State"=enum."Pause"} ("Data"), error in (no error)=w609) -> (error out=w608:errorcluster)  [unwired: 1 in, 2 out]
              }
            }
          }
          event "Stop": Value Change; User Event; Panel Close {
            # "Main"
            n131 = event-data() -> ()  [unwired: 1 in, 3 out]
            n132 = call "Control_ERD_Loop.vi"("ERD Loop"=w612, "Command (ERD Loop Control)"=ERD_Loop_Control_Command."Shutdown", "Error In"=w618) -> ("Error Out"=w617:errorcluster)  [unwired: 12 in]
            n133 = call "Control_GEA2_Loop.vi"("Command (ERD Loop Control)"=GEA2_Control_Command."Shutdown", "Error In"=w617) -> ("Error Out"=w611:errorcluster)  [unwired: 13 in]
            n134 = call "Time Delay6"("error in (no error)"=w611, "Delay Time (s)"=1.0) -> ("error out"=w613:errorcluster)  [unwired: 9 in]
          }
          event "Get Wifi Data": Value Change {
            n135 = event-data() -> ()  [unwired: 1 in, 6 out]
            n136 = call "Wifi_Data.vi"("GEA2 Reference In"=w628, "Error In"=w627) -> ("Wifi Network State"=→"Wifi Network State":string, "GEA2 Reference Out"=w623:refnum<k24>, "Mac Address"=→"Mac Address":string, "Wifi Network Name"=→"Wifi Network Name":string, "Wifi Password"=→"Wifi Password":string, "Error Out"=w626:errorcluster)  [unwired: 8 in]
          }
          event "Turn off Wifi", "Turn on Wifi": Value Change {
            w632 = T7 {"ERD Number"=61717, "Data Type"=enum."string", "Data"=""} ("ERD Read Data In")
            n137 = event-data() -> ()  [unwired: 1 in, 1 out]
            n138 = case shown="True" "Turn on Wifi" {
              tunnel: w637 -> [w660 w667]
              tunnel: w636 -> [w661 w666]
              tunnel: w632 -> [_ w665]
              tunnel: [w661 w663] -> w634
              tunnel: [w660 w664] -> w635
              tunnel: w638 -> [w659 w662]
              tunnel: [w659 w662] -> w633
              frame False {
              }
              frame True {
                n139 = Concatenate Strings("01" ("string")) -> (w678:string)
                n140 = Bundle By Name(cluster=w665, "Data"=w678) -> (w677:T7)
                n141 = Build Array(w677) -> (w668:T7[])
                n142 = call "Convert Write ERD List to Message.vi"("GEA Inputs"=w662, "Write ERD List"=w668, "Error In"=w666) -> ("GEA Message"=w672:T14, "Error Out"=w673:errorcluster)  [unwired: 11 in]
                n143 = call "GEA2MessageFormatter.vi"("Prefix(Send/Recv)"="SEND", "GEA2 Data In"=w672, "Error In"=w673) -> ("Output String"=w674:string, "Error Out"=w675:errorcluster)  [unwired: 11 in]
                n144 = call "GExplorer_Queue_GEA2.vi"("Output String"=w674, "error in (no error)"=w675) -> ("error out"=w671:errorcluster)  [unwired: 13 in]
                n145 = call "GEA2 Write ERD.vi"("GEA2 Reference In"=w667, "GEA Inputs"=w662, "Write ERD List"=w668, "Error In"=w671, "Verify ERD Response?"=FALSE) -> ("GEA2 Reference Out"=w664:refnum<k24>, "Error Out"=w663:errorcluster)  [unwired: 8 in, 1 out]
              }
            }
            n146 = case shown="True" "Turn off Wifi" {
              tunnel: w635 -> [w640 w647]
              tunnel: w634 -> [w641 w646]
              tunnel: [w641 w644] -> w629
              tunnel: [w640 w645] -> w630
              tunnel: w633 -> [_ w643]
              tunnel: w632 -> [_ w642]
              frame False {
              }
              frame True {
                n147 = Concatenate Strings("02" ("string")) -> (w658:string)
                n148 = Bundle By Name(cluster=w642, "Data"=w658) -> (w657:T7)
                n149 = Build Array(w657) -> (w648:T7[])
                n150 = call "Convert Write ERD List to Message.vi"("GEA Inputs"=w643, "Write ERD List"=w648, "Error In"=w646) -> ("GEA Message"=w652:T14, "Error Out"=w653:errorcluster)  [unwired: 11 in]
                n151 = call "GEA2MessageFormatter.vi"("Prefix(Send/Recv)"="SEND", "GEA2 Data In"=w652, "Error In"=w653) -> ("Output String"=w654:string, "Error Out"=w655:errorcluster)  [unwired: 11 in]
                n152 = call "GExplorer_Queue_GEA2.vi"("Output String"=w654, "error in (no error)"=w655) -> ("error out"=w651:errorcluster)  [unwired: 13 in]
                n153 = call "GEA2 Write ERD.vi"("GEA2 Reference In"=w647, "GEA Inputs"=w643, "Write ERD List"=w648, "Error In"=w651, "Verify ERD Response?"=FALSE) -> ("GEA2 Reference Out"=w645:refnum<k24>, "Error Out"=w644:errorcluster)  [unwired: 8 in, 1 out]
              }
            }
          }
          event "EndOfCycle": Value Change {
            n154 = event-data() -> ()  [unwired: 1 in, 1 out]
            n155 = call "GEA2 Write ERD.vi"("GEA2 Reference In"=w684, "GEA Inputs"=w681, "Write ERD List"=T7[] [{"ERD Number"=61467, "Data Type"=enum."string", "Data"="05"}], "Error In"=w683) -> ("GEA2 Reference Out"=w680:refnum<k24>, "Error Out"=w679:errorcluster)  [unwired: 9 in, 1 out]
          }
          event "Set Wifi State(ERD 6003)": Value Change {
            n156 = event-data() -> ()  [unwired: 1 in, 6 out]
            n157 = case shown="\"0 - OFF\", Default" "Wifi State" {
              tunnel: ["00" "01" "02" "03" "04" "05" "06" "FF"] -> w691
              frame "0 - OFF", Default {
              }
              frame "1 - App Mode" {
              }
              frame "2 - Connecting" {
              }
              frame "3 - Connected" {
              }
              frame "4 - Connected Off" {
              }
              frame "5 - Scanning" {
              }
              frame "6 - Reconnecting" {
              }
              frame "255 - Invalid" {
              }
            }
            n158 = case shown="True" "Set Wifi State(ERD 6003)" {
              tunnel: w687 -> [w692 w697]
              tunnel: w688 -> [w693 w701]
              tunnel: [w693 w699] -> w686
              tunnel: [w692 w700] -> w685
              tunnel: w691 -> [_ w698]
              frame False {
              }
              frame True {
                w694 = T11 {"Source"=228, "Destination"=191} ("GEA Inputs")
                n159 = Concatenate Strings(w698) -> (w710:string)
                n160 = Bundle By Name(cluster=T7 {"ERD Number"=24579, "Data Type"=enum."string", "Data"=""} ("ERD Write Data In"), "Data"=w710) -> (w709:T7)
                n161 = Build Array(w709) -> (w695:T7[])
                n162 = call "Convert Write ERD List to Message.vi"("GEA Inputs"=w694, "Write ERD List"=w695, "Error In"=w701) -> ("GEA Message"=w705:T14, "Error Out"=w706:errorcluster)  [unwired: 11 in]
                n163 = call "GEA2MessageFormatter.vi"("Prefix(Send/Recv)"="SEND", "GEA2 Data In"=w705, "Error In"=w706) -> ("Output String"=w707:string, "Error Out"=w708:errorcluster)  [unwired: 11 in]
                n164 = call "GExplorer_Queue_GEA2.vi"("Output String"=w707, "error in (no error)"=w708) -> ("error out"=w704:errorcluster)  [unwired: 13 in]
                n165 = call "GEA2 Write ERD.vi"("GEA2 Reference In"=w697, "GEA Inputs"=w694, "Write ERD List"=w695, "Error In"=w704, "Verify ERD Response?"=FALSE) -> ("GEA2 Reference Out"=w700:refnum<k24>, "Error Out"=w699:errorcluster)  [unwired: 8 in, 1 out]
              }
            }
          }
        }
        n166 = call "Error_Control.vi"("Error In"=w330) -> ("Error Out"=w332:errorcluster)  [unwired: 14 in]
      }
      n167 = while "Periodic ERD Query Loop" {
        shift-right: [w116] -> w65
        shift-left: w29 -> [w118]
        tunnel: w52 -> [w119]
        shift-right: [w111] -> _
        shift-left: w66 -> [w112]
        shift-right: [w106] -> _
        shift-left: _ -> [w105]
        tunnel: w27 -> [w104]
        tunnel: [w103] -> w63
        shift-right: [w102] -> _
        shift-left: T25 {"Version"={"Build Number"="", "Build Hash "="", "Application Version"="", "Parametric Version"="", "UI App Version"=""}, "Personality Set"=0, "CSV File String Arrays"={"ERD Number Array"=[], "ERD Name Array"=[], "ERD Converted String Data"=[]}, "Fault Table Array "=[], "ERD_Always Show"={"Machine State"="", "Cycle Selected"="", "Cycle Engine State"="", "Cycle Count"=0, "Temp Level"="", "Dryness Level"="", "Time Level"="", "Delay Time (min)"=0, "Sub-Cycle"="", "Cycle Name"="", "Tune ID"="", "Restr Detect Status"="", "Load Size by Contact"="", "Load Size by Temp"="", "EOC Reason"="", "Reset Count"="", "Dampness State"="", "Stator RL3"=FALSE, "TBD5"=FALSE, "TBD6"=FALSE, "Water Pump"=FALSE, "Stator RL2"=FALSE, "Cool Down Status"="", "TBD8"=FALSE, "TBD9"=FALSE, "TBD10"=FALSE, "TBD11"=FALSE, "TBD7"=FALSE, "Stator RL1"=FALSE, "IHC TimeSeconds"=0, "ECT TimeSeconds "=0, "Load Size by Ag"="", "Dry Load Detection"=""}, "UI LEDS"={"Led 1"=FALSE, "Led 2"=FALSE, "Led 3"=FALSE, "Led 4"=FALSE, "Led 5"=FALSE, "Led 6"=FALSE}, "Boot Loader Version"={"UI BL Version"="", "MC BL Version"=""}} ("All_Bundled_Data_Brass") -> [w101]
        shift-right: [w99] -> _
        shift-left: _ -> [w98]
        shift-right: [w97] -> _
        shift-left: _ -> [w96]
        shift-right: [w94] -> _
        shift-left: _ -> [w93]
        stop <- w115 stop-if-true
        # "Todas los pasos de esta ciclo se ejecutan una ves al iniciar el programa"
        # "ERD Loop"
        n168 = Dequeue Element(queue=w119, timeout in ms (-1)=0, error in (no error)=w118) -> (element=w108:T30, timed out?=w100:bool, error out=w117:errorcluster)  [unwired: 1 out]
        n169 = Unbundle By Name(w108) -> ("State"=w113:T36)
        n170 = Select(t=w112, s=w100, f=w113) -> (s? t:f=w95:T36)
        "State" <- w95
        n171 = call "FGV_GEA2_Ref.vi"("Action"=enum16{"Set Ref", "Get Ref"}."Get Ref", "Error In"=w117) -> ("GEA2 Reference Out"=w107:refnum<k24>, "Error Out"=w110:errorcluster)  [unwired: 12 in]
        n172 = case shown="\"Init\", Default" w95 {
          tunnel: w110 -> [w131 w141 w166 w189 w211 w239 w267 w276]
          tunnel: [w125 w135 w163 w190 w211 w236 w267 w276] -> w114
          tunnel: [_ _ _ _ _ _ _ TRUE] -> w115
          tunnel: [ERD_Loop_States."Get Version" ("State") ERD_Loop_States."Build ERD Read List" ("State") ERD_Loop_States."Read ERDs" ("State") ERD_Loop_States."Update UI" ("State") ERD_Loop_States."Log Data" ("State") ERD_Loop_States."Pause" ("t") ERD_Loop_States."Read ERDs" ("State") ERD_Loop_States."Shutdown" ("State")] -> w111
          tunnel: w107 -> [_ w140 _ w185 _ _ _ _]
          tunnel: [w129 w149 w165 w186 w215 w243 w265 w273] -> w106
          tunnel: w105 -> [w129 w149 _ w186 w215 w243 w265 w273]
          tunnel: w104 -> [w128 w148 w162 w200 w212 w224 w264 w272]
          tunnel: [w128 w148 w162 w200 w212 w242 w264 w272] -> w103
          tunnel: [T25 {"Version"={"Build Number"="", "Build Hash "="", "Application Version"="", "Parametric Version"="", "UI App Version"=""}, "Personality Set"=0, "CSV File String Arrays"={"ERD Number Array"=[], "ERD Name Array"=[], "ERD Converted String Data"=[]}, "Fault Table Array "=[], "ERD_Always Show"={"Machine State"="", "Cycle Selected"="", "Cycle Engine State"="", "Cycle Count"=0, "Temp Level"="", "Dryness Level"="", "Time Level"="", "Delay Time (min)"=0, "Sub-Cycle"="", "Cycle Name"="", "Tune ID"="", "Restr Detect Status"="", "Load Size by Contact"="", "Load Size by Temp"="", "EOC Reason"="", "Reset Count"="", "Dampness State"="", "Stator RL3"=FALSE, "TBD5"=FALSE, "TBD6"=FALSE, "Water Pump"=FALSE, "Stator RL2"=FALSE, "Cool Down Status"="", "TBD8"=FALSE, "TBD9"=FALSE, "TBD10"=FALSE, "TBD11"=FALSE, "TBD7"=FALSE, "Stator RL1"=FALSE, "IHC TimeSeconds"=0, "ECT TimeSeconds "=0, "Load Size by Ag"="", "Dry Load Detection"=""}, "UI LEDS"={"Led 1"=FALSE, "Led 2"=FALSE, "Led 3"=FALSE, "Led 4"=FALSE, "Led 5"=FALSE, "Led 6"=FALSE}, "Boot Loader Version"={"UI BL Version"="", "MC BL Version"=""}} ("All_Bundled_Data_Brass") w134 w161 w192 w213 w222 w263 w271] -> w102
          tunnel: w101 -> [_ w139 w161 w195 w213 w222 w263 w271]
          tunnel: [w122 w137 w154 w193 w210 w227 w262 w270] -> w99
          tunnel: w98 -> [w122 w137 _ w193 w210 w227 w262 w270]
          tunnel: [w124 w147 w160 w198 w209 w226 w261 w269] -> w97
          tunnel: w96 -> [w124 w147 w160 w197 w209 w226 w261 w269]
          tunnel: [w121 w132 w155 w178 w205 w217 w259 w268] -> w94
          tunnel: w93 -> [w121 w132 _ w178 w205 w217 w259 w268]
          frame "Init", Default {
            # "Set Write Header\nFGV to True"
            n173 = call "Write_Header_FGV.vi"("Write Header ? In"=TRUE, "Action"=enum16{"Get", "Set"}."Set", "Error In"=w131) -> ("Error Out"=w125:errorcluster)  [unwired: 11 in, 1 out]
          }
          frame "Get Version" {
            # "MC"
            n174 = call "GEA3 Read ERD (Rev 2 API) Multiple Messages.vi"("GEA2 Reference In"=w140, "Retry Count"=1 ("# of Iterations (Should be 2 except JL)"), "Read Timeout (ms)"=u32 250, "GEA Inputs"=cluster{"Source":u8, "Destination":u8} {"Source"=228, "Destination"=192}, "Read ERD List"=T6[] [{"ERD Number"=127, "Data Type"=enum."string"}, {"ERD Number"=49, "Data Type"=enum."string"}, {"ERD Number"=57, "Data Type"=enum."string"}, {"ERD Number"=58, "Data Type"=enum."string"}, {"ERD Number"=59, "Data Type"=enum."string"}] ("Read ERD List MC"), "Error In"=w141, "Verify ERD Response?"=FALSE) -> ("ERD Data Out"=w138:cluster{"ERD Number":u16, "Data":string}[], "Error Out"=w136:errorcluster)  [unwired: 5 in, 2 out]
            n175 = call "Convert_ERDs_Version_ARG.vi"("New Header?"=TRUE, "ERD Name"=w137, "All_Bundled_Data_Brass"=w139, "Array"=w138, "Error In"=w136) -> ("All_Bundled_Data_Brass 2"=w134:T25, "Error Out"=w135:errorcluster)  [unwired: 9 in]
          }
          frame "Build ERD Read List" {
            n176 = Build Array (concatenate)("ERD Default List", "ERD's List Ticket Testing") -> (w159:T20)
            n177 = for {
              shift-right: [w169] -> w155
              shift-left: 0 -> [w168]
              tunnel: "ERD Default List" -> [w167] mode=indexing
              n178 = Unbundle By Name(w167) -> ("Boolean"=w170:bool)
              n179 = case shown="True" w170 {
                tunnel: [w171 w173] -> w169
                tunnel: w168 -> [w171 w172]
                frame False {
                }
                frame True {
                  n180 = Increment(x=w172) -> (x+1=w173:i32)
                }
              }
            }
            n181 = call "ERD_Read_List_Builder.vi"("ERD Read List ALL"=w159, "Error In"=w166) -> ("Read ERD List"=w165:T6[], "ERD Name"=w154:string[], "Error Out"=w163:errorcluster)  [unwired: 15 in]
            n182 = Array Size(array="ERD Default List") -> (size(s)=w153:i32)
            n183 = Array Subset(array=w154, index=w153) -> (w152:string[])  [unwired: 1 in]
            n184 = property on="ERD's de Usuario" class="Clust (strict)"() -> ("Controls[]"=w157:refnum<vi>[])  [unwired: 2 in, 2 out]
            n185 = for {
              tunnel: w157 -> [w175] mode=indexing
              tunnel: w152 -> [w174] mode=indexing
              n186 = property class="Ctl"(reference=w175, "Caption.Visible"=TRUE, "Label.Visible"=FALSE, "Caption.Text"=w174) -> ()  [unwired: 1 in, 2 out]
            }
          }
          frame "Read ERDs" {
            n187 = call "Add Version Data to User ERD list.vi"(".NET Refnum in"=w185, "# of Iterations (Should be 2 except JL)"=1, "Read ERD List MC"=w186, "error in (no error)"=w189, "#ERDs per message"=20) -> ("ERD Data Out out"=w179:T9[], "error out"=w188:errorcluster)  [unwired: 9 in]
            n188 = call "Write_Header_FGV.vi"("Action"=enum16{"Get", "Set"}."Get", "Error In"=w188) -> ("Write Header ? Out"=w191:bool, "Error Out"=w194:errorcluster)  [unwired: 12 in]
            n189 = Tick Count (ms)() -> (millisecond timer value=w198:u32)
            n190 = call "Convert_ERDs_ARG.vi"("New Header?"=w191, "ERD Name"=w193, "All_Bundled_Data_Brass"=w195, "Array"=w179, "Error In"=w194) -> ("All_ERD_Data_Bundled_Brass"=w192:T25, "Error Out"=w190:errorcluster)  [unwired: 9 in]
            n191 = Subtract(x=w198, y=w197) -> (x-y=→"Rate":u32)
            n192 = Array Subset(array=w179, index=w178) -> (w180:T9[])  [unwired: 1 in]
            n193 = for {
              tunnel: [w203] -> w182 mode=indexing
              tunnel: w180 -> [w202] mode=indexing
              n194 = Unbundle By Name(w202) -> ("Data"=w203:string)
            }
            n195 = Build Array (concatenate)(w182) -> (w183:string[])
            n196 = Array To Cluster(array=w183) -> (cluster=→"ERD's de Usuario":T12)
          }
          frame "Update UI" {
            n197 = Unbundle By Name(w213) -> ("Boot Loader Version"=→"Boot Loader Version":T10, "Version"=→"Version":T5, "Personality Set"=→"Personality Set":u8, "ERD_Always Show"=→"ERD_Always Show":T2, "UI LEDS"=→"UI LEDS":T1)
          }
          frame "Log Data" {
            # "TimeStamp"
            # "Append With Fault Log Data"
            n198 = Unbundle By Name(w222) -> ("CSV File String Arrays.ERD Name Array"=w241:string[], "CSV File String Arrays.ERD Number Array"=w218:string[], "CSV File String Arrays.ERD Converted String Data"=w225:string[])
            n199 = call "Write_Header_FGV.vi"("Action"=enum16{"Get", "Set"}."Get", "Error In"=w239) -> ("Write Header ? Out"=w228:bool, "Error Out"=w234:errorcluster)  [unwired: 12 in]
            n200 = case shown="True" w228 {
              tunnel: w241 -> [w246 _]
              tunnel: w224 -> [w252 w258]
              tunnel: [w251 w258] -> w223
              tunnel: w222 -> [w244 _]
              tunnel: w218 -> [w245 _]
              frame True {
                # "Write Header"
                n201 = call "Build_Header_ARG.vi"("All_Bundled_Data_Brass"=w244, "ERD Number Array In"=w245, "ERD Name Array In"=w246) -> ("ERD Name Array out 2"=w247:string[][])  [unwired: 8 in]
                n202 = Array Size(array=w247) -> (size(s)=w250:i32[])
                n203 = Index Array(array=w250, index=1) -> (element=w248:i32)
                n204 = for {
                  N: w248 -> [_]
                  tunnel: w252 -> [w257]
                  tunnel: [w256] -> w251
                  tunnel: w247 -> [w255]
                  i -> [w254]
                  n205 = Index Array(array=w255, index (row)=w254) -> (element=w253:string[])  [unwired: 1 in]
                  n206 = call "Write _To_CSV_File.vi"("Refnum In"=w257, "ERD Name"=w253) -> ("Refnum Out"=w256:refnum<file>)  [unwired: 15 in, 2 out]
                }
              }
              frame False {
              }
            }
            n207 = call "TimeStamp to String Array.vi"("String Array In"=w225) -> ("String Array Out"=w221:string[])  [unwired: 10 in]
            n208 = Unbundle By Name(w222) -> ("Fault Table Array"=w230:T27)
            n209 = call "Faults_To_String_Array.vi"("Write Header ?"=w228, "Fault Table Entry"=w230, "Error In"=w234) -> ("Fault Header String Array"=w220:string[], "Fault ERD Number String Array"=w219:string[], "Fault Data String Array"=w233:string[], "Error Out"=w231:errorcluster)  [unwired: 13 in]
            n210 = Insert Into Array(array=w221, new element=w233) -> (w232:string[])  [unwired: 1 in]
            n211 = call "Write _To_CSV_File.vi"("Refnum In"=w223, "ERD Name"=w220, "ERD Number"=w219, "ERD Data"=w232, "Error In"=w231) -> ("Refnum Out"=w242:refnum<file>, "Error Out"=w237:errorcluster)  [unwired: 12 in, 1 out]
            n212 = call "Write_Header_FGV.vi"("Write Header ? In"=FALSE, "Action"=enum16{"Get", "Set"}."Set", "Error In"=w237) -> ("Error Out"=w236:errorcluster)  [unwired: 11 in, 1 out]
          }
          frame "Pause" {
            n213 = Wait Until Next ms Multiple(millisecond multiple="Pause(mls)") -> ()  [unwired: 1 out]
          }
          frame "Shutdown" {
          }
        }
        n214 = call "Error_Control.vi"("Error In"=w114) -> ("Error Out"=w116:errorcluster)  [unwired: 14 in]
      }
      n215 = while "GEA2 Display Loop" {
        tunnel: w51 -> [w286]
        shift-right: [w283] -> _
        shift-left: "" -> [w289]
        shift-right: [w285] -> w82
        shift-left: w57 -> [w293]
        tunnel: w56 -> [w279]
        tunnel: [w277] -> w54
        stop <- w287 stop-if-true
        # "Mensajes de los comandos enviados"
        # "GEA2 Display Loop"
        n216 = Dequeue Element(queue=w286, error in (no error)=w293) -> (element=w292:T32, error out=w288:errorcluster)  [unwired: 1 in, 2 out]
        n217 = Unbundle By Name(w292) -> ("Data"=w290:variant, "State"=w291:enum16{"Add to Log", "Clear", "Shutdown"})
        n218 = case shown="\"Add to Log\", Default" w291 {
          tunnel: w290 -> [w304 _ _]
          tunnel: w289 -> [w307 w312 _]
          tunnel: [w306 w312 ""] -> w284
          tunnel: w288 -> [w305 w313 w317]
          tunnel: [w302 w313 w317] -> w280
          tunnel: [FALSE TRUE FALSE] -> w287
          tunnel: [w294 _ _] -> w278
          frame "Add to Log", Default {
            n219 = Variant To Data(error in=w305, type="", Variant=w304) -> (data=w296:string, error out=w302:errorcluster)
            n220 = String Subset(string=w296, offset (0)=22, length (rest)=7 ("length (rest)")) -> (substring=w297:string)
            n221 = Equal?(x="SEND E4", y=w297) -> (x = y?=w295:bool)
            n222 = case shown="True" w295 {
              tunnel: w307 -> [w310 w311]
              tunnel: [w309 w311] -> w306
              tunnel: w296 -> [w308 _]
              tunnel: [w308 _] -> w294
              frame False {
                n223 = Concatenate Strings(w308, w310) -> (w309:string)
              }
              frame True {
              }
            }
          }
          frame "Shutdown" {
          }
          frame "Clear" {
          }
        }
        "GEA2 Log" <- w284
        n224 = call "Write _To_TXT_File.vi"("refnum"=w279, "text"=w278, "error in"=w280) -> ("refnum out"=w277:refnum<file>, "error out"=w281:errorcluster)  [unwired: 10 in, 1 out]
        n225 = String Subset(string=w284, length (rest)="GEA2 Log Length") -> (substring=w283:string)  [unwired: 1 in]
        n226 = call "Error_Control.vi"("Error In"=w281) -> ("Error Out"=w285:errorcluster)  [unwired: 14 in]
      }
      n227 = call "GEA2 Stop.vi"("GEA2 Reference In"=w91, "Error In"=w92) -> ("Error Out"=w24:errorcluster)  [unwired: 13 in]
      n228 = Close File(refnum=w54, error in=w82) -> (error out=w55:errorcluster)  [unwired: 1 out]
      n229 = Close File(refnum=w63, error in=w65) -> (error out=w64:errorcluster)  [unwired: 1 out]
      n230 = Merge Errors(w64, w55, w24) -> (w80:errorcluster)
      n231 = Obtain Queue(name (unnamed)="Continuous Send", element data type=Cont_Send_States."Run" ("State")) -> (queue out=w62:refnum<queue>, error out=w61:errorcluster)  [unwired: 3 in, 1 out]
      n232 = Obtain Queue(name (unnamed)="ERD Loop", element data type=T30 {"Data"=variant, "State"=enum."Read ERDs"} ("Data"), error in (no error)=w80) -> (queue out=w84:refnum<queue>, error out=w83:errorcluster)  [unwired: 2 in, 1 out]
      n233 = Obtain Queue(name (unnamed)="GEA2", element data type=T32 {"Data"=variant, "State"=enum."Add to Log"} ("Data"), error in (no error)=w80) -> (queue out=w90:refnum<queue>, error out=w89:errorcluster)  [unwired: 2 in, 1 out]
      n234 = Release Queue(queue=w62, error in (no error)=w61) -> (error out=w60:errorcluster)  [unwired: 1 in, 2 out]
      n235 = Release Queue(queue=w84, error in (no error)=w83) -> (error out=w78:errorcluster)  [unwired: 1 in, 2 out]
      n236 = Release Queue(queue=w90, error in (no error)=w89) -> (error out=w79:errorcluster)  [unwired: 1 in, 2 out]
      n237 = Merge Errors(w60, w78, w79) -> (w77:errorcluster)
      n238 = call "Error_Control.vi"("Command (Handle Errors)"=Error_Command."Report Errors", "Error In"=w77) -> ("Error Out"=w76:errorcluster)  [unwired: 13 in]
    }
    frame Error {
    }
  }
  n239 = property on="ERD's de Usuario" class="Clust (strict)"(error in=w2) -> (error out=w3:errorcluster, "Controls[]"=w5:refnum<vi>[])  [unwired: 1 in, 1 out]
  n240 = for {
    tunnel: w5 -> [w723] mode=indexing
    tunnel: string[] ["User 1", "User 2", "User 3", "User 4", "User 5", "User 6", "User 7", "User 8", "User 9", "User 10"] -> [w722] mode=indexing
    tunnel: w3 -> [w721]
    tunnel: [w720] -> w1
    n241 = property class="Ctl"(reference=w723, error in=w721, "Caption.Visible"=TRUE, "Label.Visible"=FALSE, "Caption.Text"=w722) -> (error out=w720:errorcluster)  [unwired: 1 out]
  }
  n242 = call <vilib>:"Simple Error Handler.vi"("error in (no error)"=w1) -> ("error out"=→"Error Out":errorcluster)  [unwired: 4 in, 4 out]
